vi "MonoVu.vi"() -> ()   [LabVIEW 2020]
doc: "Sequence Program with the Message Handling Queue (MHQ) for the National High Magnetic Field Laboratory in Tallahassee, Florida. \nOnce you understand how the programs works, you should be able to modify this program easily. If you have any questions, contact Minseong Lee(ml10k@my.fsu.edu), who first made this program in June, 2015."
uses:
  <vilib>/printing/OpenHTMLReport.llb/Open HTML Report in Browser (String).vi
  <vilib>/Utility/NIReport.llb/NI_ReportGenerationCore.lvlib
panel:
  out "error out":errorcluster
  in  "error\ncheck":bool
  out "macro line":i32
  in  "exec window":bool caption="command window"
  in  "loop stop":bool
  in  "looped command interval (ms)":u32=100
  in  "wait (ms)":u32
  in  "reset error indicator":bool
  out "Error/\nwarning?":bool
  in  "override command error":bool
  in  "platform":u16(ring) items=["Mac", "PC"]
  out "execution count":i32=1
  in  "sequence utility":bool caption="seq\n utility"
  out "macro cmd no":i32=3
  in  "go to \ncurrent":bool
  in  "help":bool caption="Help"
  in  "Magnet PS":u16(ring)=4 items=["Resistive Magnet", "SCM2", "SCM1", "Generic SC power supply", "PPMS"]
  out "Buffer Edit":string[](array[string])
  out "Path":path=path "/Users/Shared/NML Data Acquisition/Monovu/sequence templates/Examples.txt"
  out "Buffer History":string[](array[string])
  in  "NML Data Acquisition VI":string(combo)="NML Data Acquisition-New.vi"
  in  "Skip Button":bool caption="Skip"
  out "latest error":errorcluster={"status"=TRUE, "code"=1004, "source"="Open VI Reference in Run_VI.vi->MonoVu.vi<APPEND>\nTo load a VI into memory with the Open VI Reference function, a path must be wired for the VI Path input.\n\nVI Name: <b>dsfasdf.vdsafisdaf</b>"}
  in  "error in (no error)":errorcluster
  in  "New Button":bool caption="New"
  in  "Program Stop":bool caption="Program \nStop"
  out "Sequence Status":string="Idle"
  in  "Commands":string(tree)="Set Field"
  in  "Sequence":i32[](listbox)=[16] caption="Sequence*"
  in  "Save Button":bool caption="Save"
  in  "Sequence_Stop":bool caption="Stop"
  in  "Pause Button":bool caption="Pause"
  in  "Run Sequence":bool caption="Run"
  in  "Save As Button":bool caption="Save As"
  out "Cursor Position":i32=16
  out "Current Line":i32
  in  "Open Button":bool caption="Open"
  # "Wait between each execution of command.\ne.g.  if the value is 10, and the command is \n'Wait for Temperature', it checks the temperature every 10 msec. It also forces pause between commands."
  # "(see logbook for previous errors)"
  # "(bypass command syntax error)"
  # "1. Each comand in the sequence line is executed repeatedly until a 'go to next line' command is issued by itself or interrupted by the user. \n2. 'go to next line' condition is defined in the VI for each command. \n\nNote\n(1) For commands with timed or conditioned wait, 'go to next line' command will be issued when the certain condition is met.\n(2) For non-wait command (send command to instruments or VI without waiting response), 'go to next line' is executed automatically.\n(3) For example, 'wait for temperature command' executes repeatedly until the temperature condition is met. The visa reference will be open and closed every time it is executed.\n** Exception: 'Wait for VI value' uses a loop to use the VI reference. The loop condition has to be programmatically reset for the user intervention (skip, pause, stop) accordingly."
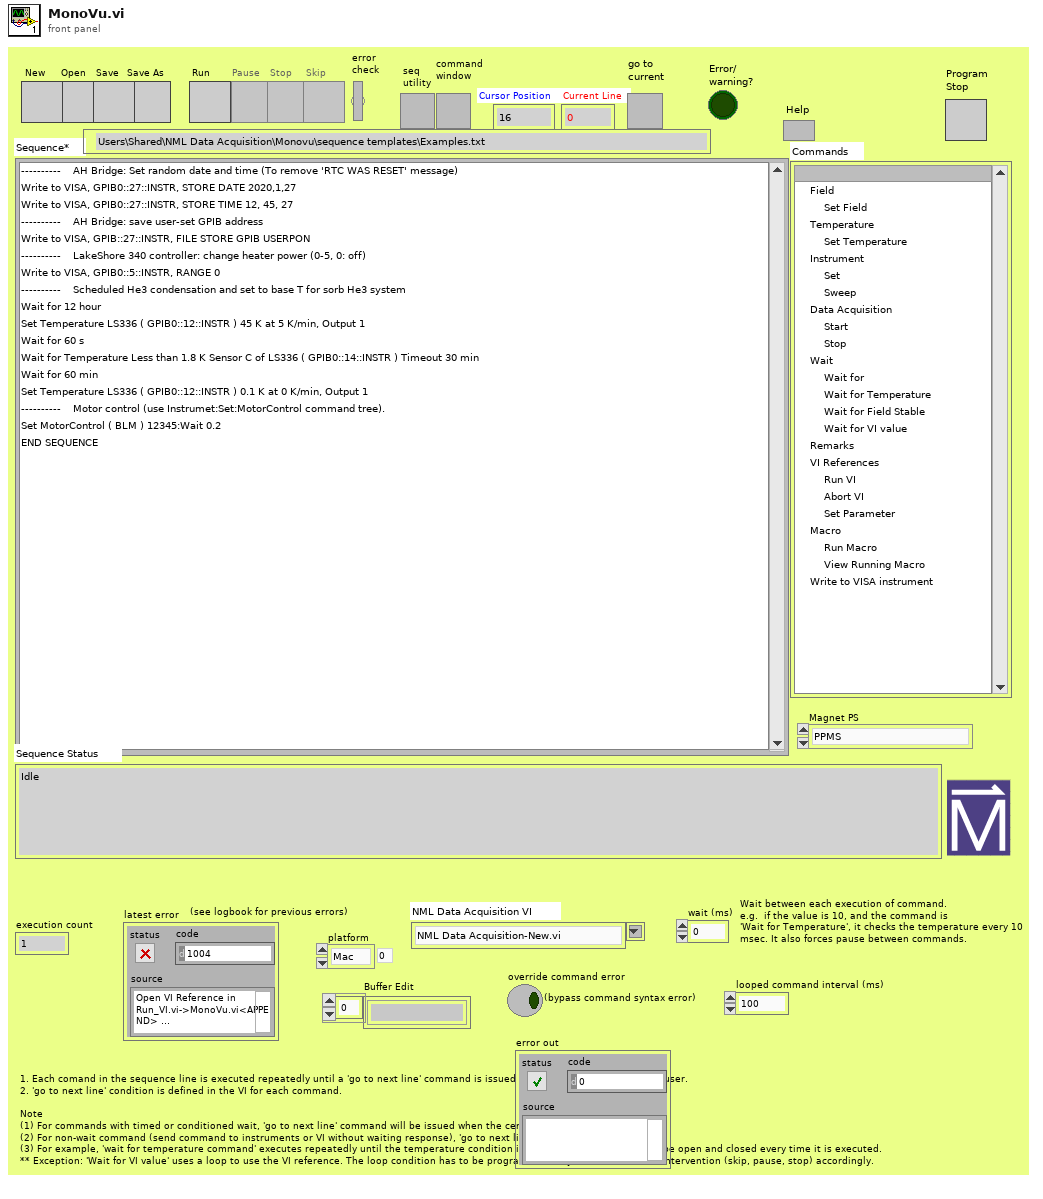
[diagram p1: front panel]
types:
  T1 = cluster{"Sequence_Run":refnum<vi>, "Sequence_Pause":refnum<vi>, "Sequence_Stop":refnum<vi>, "Sequence_Skip":refnum<vi>, "Program Stop":refnum<vi>, "Sequence":refnum<vi>, "NML Data Acquisition VI":refnum<vi>}
  T2 = cluster{"number of line":i32, "Signal":bool, "Command":string, "Sequence Reference":refnum<vi>, "Add or modification":bool}
  T3 = cluster{"No. of command":i32, "Parameters":string[], "Address":refnum<visa-resource-name>, "Boolean":bool, "No. of line":i32, "Initial Time":timestamp, "Current Time":timestamp, "Status":string, "Sequence Ref.":refnum<vi>, "Temp_Check":i32, "Sequence_History":string, "Subsequence":string[]}
  T4 = typedef "Command_Message.ctl" = cluster{"No. of command":i32, "Parameters":string[], "Address":refnum<visa-resource-name>, "Boolean":bool, "No. of line":i32, "Initial Time":timestamp, "Current Time":timestamp, "Status":string, "Sequence Ref.":refnum<vi>, "Temp check":i32, "Sequence_History":string, "Subsequence":string[]}
  T5 = typedef "Button_Reference.ctl" = cluster{"Sequence_Run":refnum<vi>, "Sequence_Pause":refnum<vi>, "Sequence_Stop":refnum<vi>, "Sequence_Skip":refnum<vi>, "Program Stop":refnum<vi>, "Sequence":refnum<vi>, "NML Data Acquisition VI":refnum<vi>}
  T6 = typedef "Command_Queue.ctl" = refnum<queue>
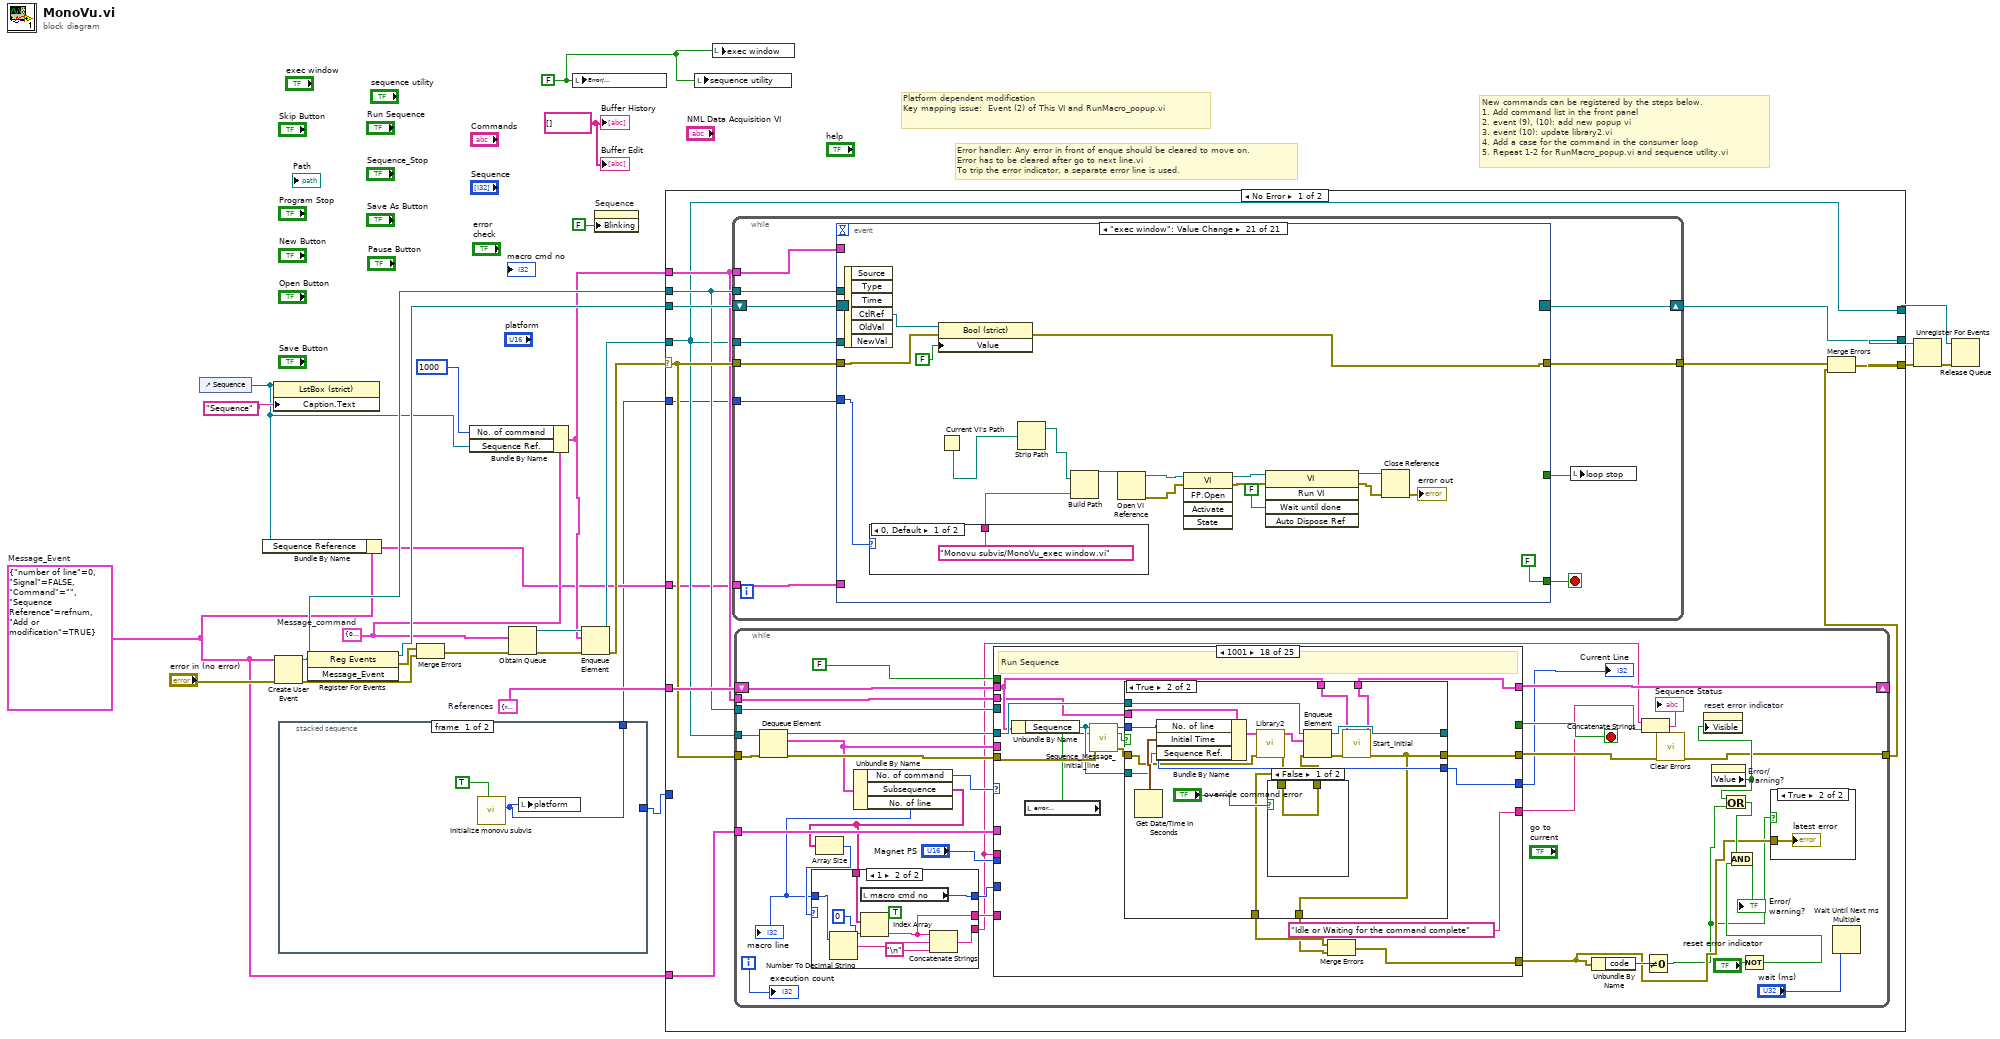
[diagram p0: block diagram]
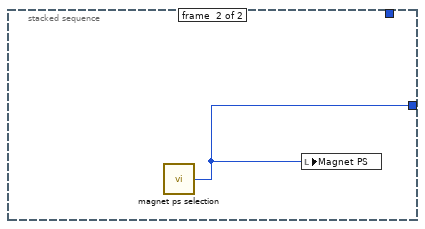
[diagram p2: hidden frame]
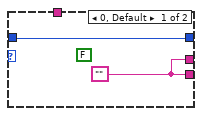
[diagram p4: hidden frame]
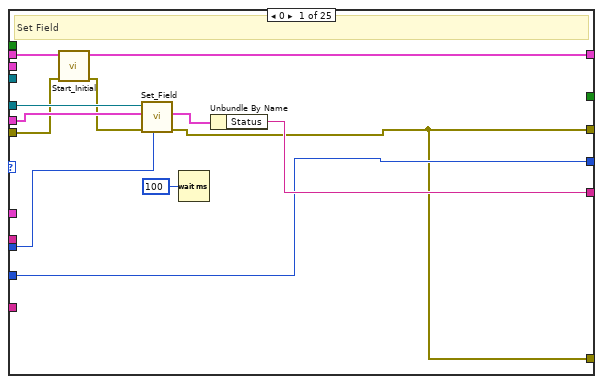
[diagram p5: hidden frame]
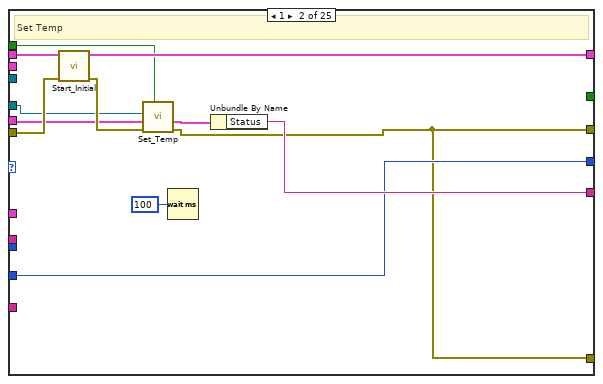
[diagram p6: hidden frame]
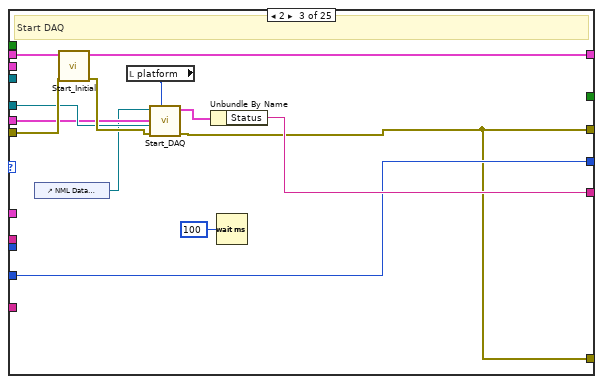
[diagram p7: hidden frame]
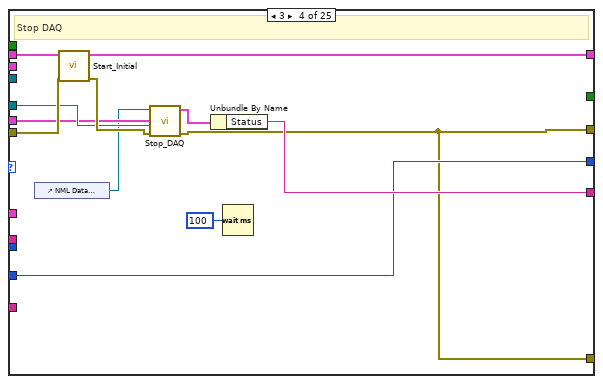
[diagram p8: hidden frame]
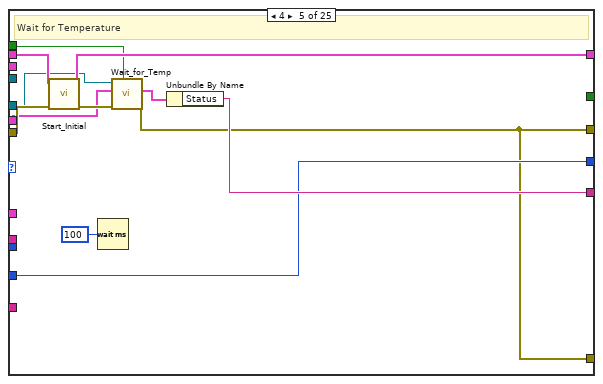
[diagram p9: hidden frame]
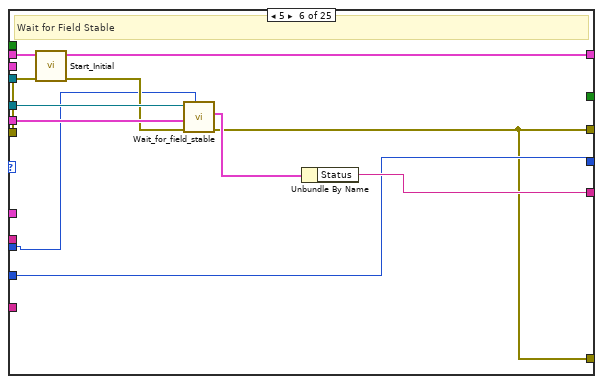
[diagram p10: hidden frame]
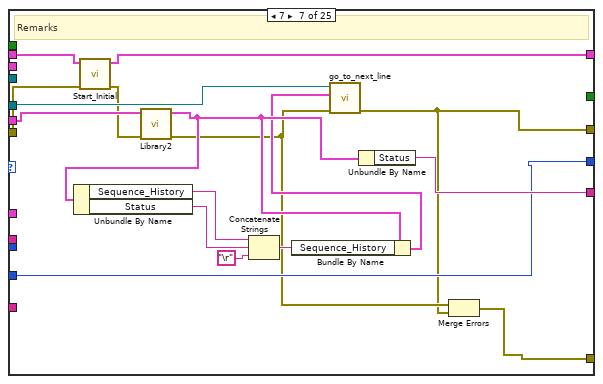
[diagram p11: hidden frame]
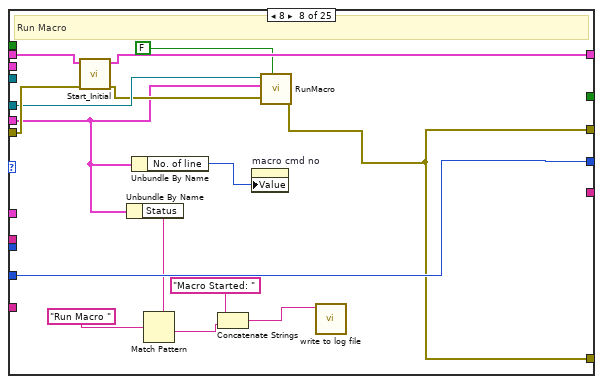
[diagram p12: hidden frame]
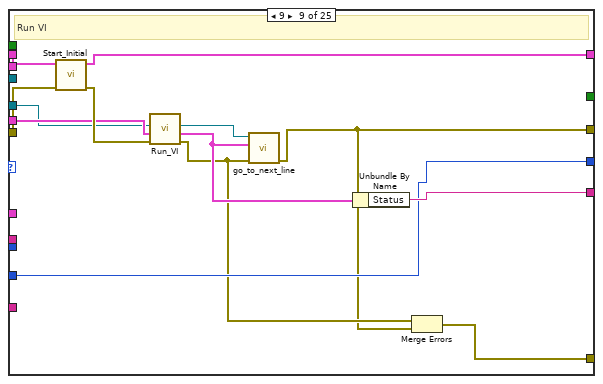
[diagram p13: hidden frame]
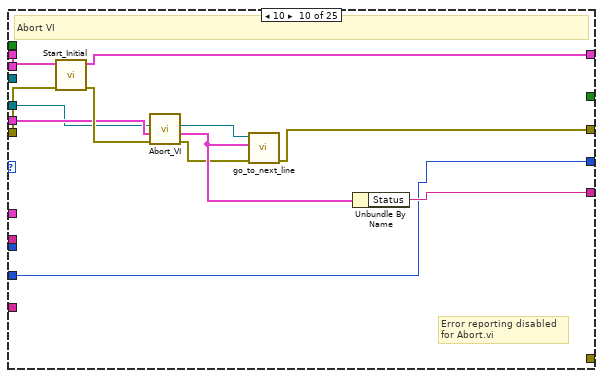
[diagram p14: hidden frame]
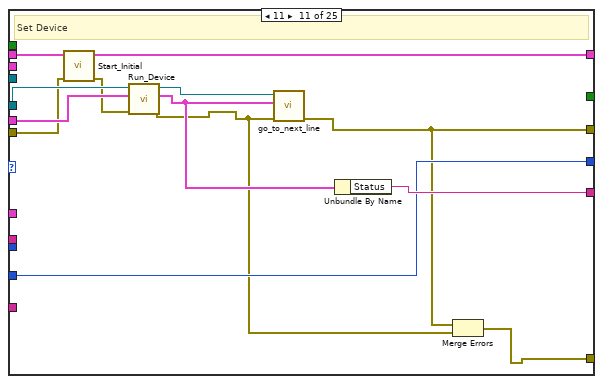
[diagram p15: hidden frame]
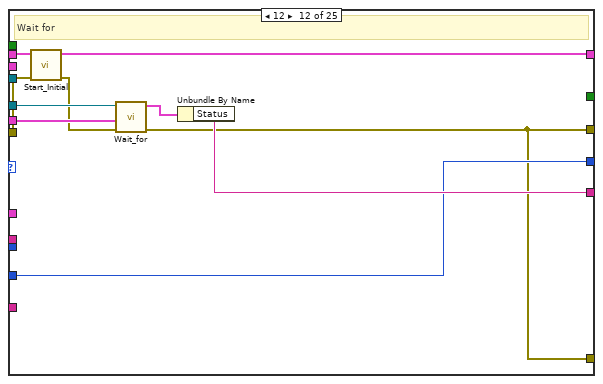
[diagram p16: hidden frame]
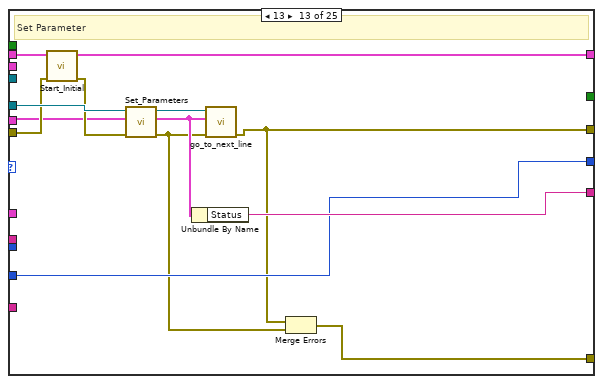
[diagram p17: hidden frame]
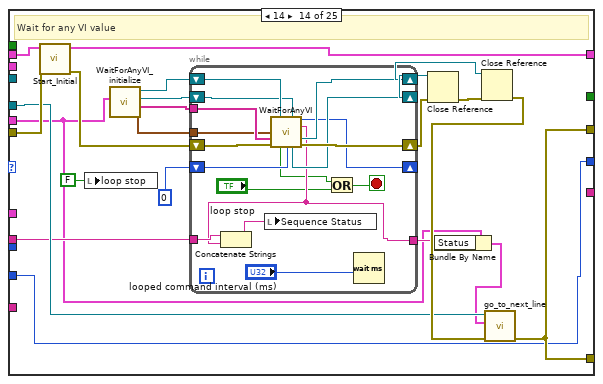
[diagram p18: hidden frame]
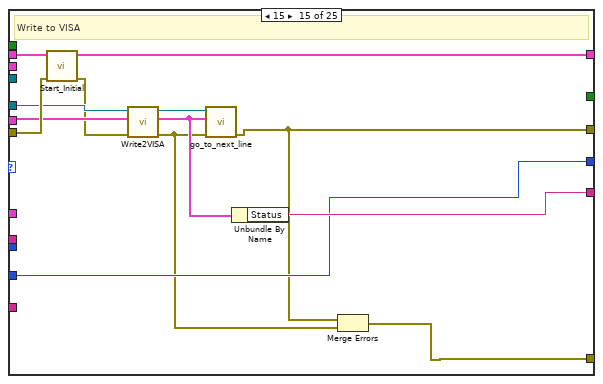
[diagram p19: hidden frame]
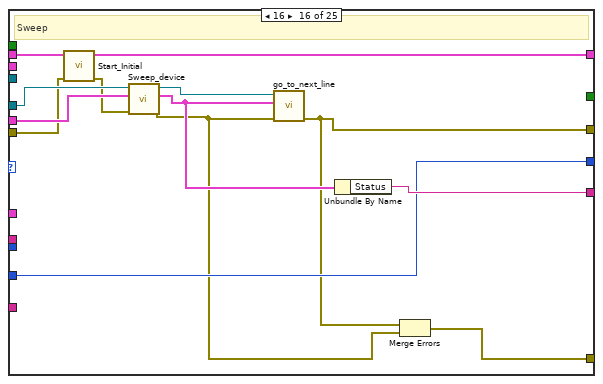
[diagram p20: hidden frame]
diagram:
  w2 = FALSE ("Error?")
  w17 = T1 {"Sequence_Run"=refnum, "Sequence_Pause"=refnum, "Sequence_Stop"=refnum, "Sequence_Skip"=refnum, "Program Stop"=refnum, "Sequence"=refnum, "NML Data Acquisition VI"=refnum}  # References
  w5 = string[] []
  w11 = T2 {"number of line"=0, "Signal"=FALSE, "Command"="", "Sequence Reference"=refnum, "Add or modification"=TRUE}  # Message_Event
  w18 = T3 {"No. of command"=0, "Parameters"=[], "Address"="", "Boolean"=TRUE, "No. of line"=0, "Initial Time"=timestamp(0 s since 1904-01-01), "Current Time"=timestamp(0 s since 1904-01-01), "Status"="", "Sequence Ref."=refnum, "Temp_Check"=0, "Sequence_History"="", "Subsequence"=[]}  # Message_command
  # "Error handler: Any error in front of enque should be cleared to move on.\nError has to be cleared after go to next line.vi\nTo trip the error indicator, a separate error line is used."
  # "Platform dependent modification\nKey mapping issue:  Event (2) of This VI and RunMacro_popup.vi"
  # "New commands can be registered by the steps below.\n1. Add command list in the front panel\n2. event (9), (10): add new popup vi\n3. event (10): update library2.vi \n4. Add a case for the command in the consumer loop\n5. Repeat 1-2 for RunMacro_popup.vi and sequence utility.vi"
  n1 = control-ref of="Sequence"() -> (w6:refnum<vi>)
  n2 = Bundle By Name(cluster=w11, "Sequence Reference"=w6) -> (w10:T2)
  n3 = property class="LstBox (strict)"(reference=w6, "Caption.Text"="Sequence") -> ()  [unwired: 1 in, 2 out]
  n4 = Create User Event(user event datatype=w11, error in="error in (no error)") -> (user event=w23:refnum<user-event>, error out=w25:errorcluster)
  n5 = stacked-sequence {
    tunnel: [_ w30] -> w1
    tunnel: [w28 _] -> w3
    frame #0 {
      n6 = call "Initialize monovu subvis.vi"("auto detect"=TRUE) -> ("platform used"=w28:u16)  [unwired: 9 in, 1 out]
      n7 = local write "platform"(w28) -> ()
    }
    frame #1 {
      n8 = call "magnet ps selection.vi"() -> ("Magnet PS"=w30:u16)  [unwired: 1 in]
      n9 = local write "Magnet PS"(w30) -> ()
    }
  }
  n10 = register-events(w23) -> (reference out=w27:refnum<event-registration>, error out=w24:errorcluster)  [unwired: 2 in]
  n11 = Merge Errors(w24, w25) -> (w8:errorcluster)
  n12 = Bundle By Name(cluster=w18, "No. of command"=1000, "Sequence Ref."=w6) -> (w16:T3)
  n13 = Obtain Queue(element data type=w18, error in (no error)=w8) -> (queue out=w22:refnum<queue>, error out=w20:errorcluster)  [unwired: 3 in, 1 out]
  n14 = local write "Error/\nwarning?"(w2) -> ()
  n15 = Enqueue Element(queue=w22, element=w16, error in (no error)=w20) -> (queue out=w21:refnum<queue>, error out=w19:errorcluster)  [unwired: 1 in, 1 out]
  n16 = property on="Sequence" class="LstBox (strict)"("Blinking"=FALSE) -> ()  [unwired: 2 in, 2 out]
  n17 = case shown="No Error" w19 {
    selector: w19 -> [w40 w1352]
    tunnel: w21 -> [w36 w1350]
    tunnel: [w42 w1352] -> w13
    tunnel: w23 -> [w39 _]
    tunnel: w27 -> [w43 w1351]
    tunnel: w17 -> [w41 _]
    tunnel: w16 -> [w37 _]
    tunnel: w11 -> [w38 _]
    tunnel: [w36 w1350] -> w15
    tunnel: [w34 w1351] -> w14
    tunnel: w10 -> [w32 _]
    tunnel: w1 -> [_ _]
    tunnel: w3 -> [w31 _]
    frame No Error {
      n18 = while {
        tunnel: w36 -> [w481]
        tunnel: w39 -> [w480]
        tunnel: w40 -> [w479]
        tunnel: [w478] -> w35
        tunnel: w37 -> [w477]
        shift-right: [w476] -> w34
        shift-left: w43 -> [w483]
        tunnel: w32 -> [w475]
        tunnel: w31 -> [w474]
        stop <- w482 stop-if-true
        # "Event_Handler"
        n19 = event shown="[20] \"exec window\": Value Change" {
          selector: w483 -> [_ _ _ _ _ _ _ _ _ _ _ _ _ _ _ _ _ _ _ _ _]
          dyn-events: [_ _ _ _ _ _ _ _ _ _ _ _ _ _ _ _ _ _ _ _ _] -> w476
          timeout: _ -> [_ _ _ _ _ _ _ _ _ _ _ _ _ _ _ _ _ _ _ _ _]
          tunnel: [FALSE ("NewVal") FALSE ("NewVal") FALSE ("NewVal") FALSE ("NewVal") FALSE ("NewVal") FALSE ("NewVal") FALSE ("NewVal") FALSE ("NewVal") FALSE ("NewVal") FALSE ("NewVal") FALSE ("NewVal") FALSE ("NewVal") FALSE ("NewVal") FALSE ("NewVal") FALSE ("NewVal") FALSE ("NewVal") w1306 FALSE ("NewVal") TRUE ("NewVal") _ FALSE ("NewVal")] -> w482
          tunnel: w481 -> [w487 _ _ _ _ _ _ _ _ _ _ _ w1248 _ w1285 w1300 w1301 w1309 _ _ _]
          tunnel: w480 -> [w491 _ w675 w803 _ _ _ _ _ w978 w1107 _ _ _ _ _ _ _ _ _ _]
          tunnel: w479 -> [w490 w511 w676 w805 w835 w873 w887 w915 w942 w980 w1116 w1237 w1247 _ w1283 w1299 w1302 w1310 w1316 w1325 w1345]
          tunnel: [w486 w510 w674 w804 w834 w871 w886 w914 w941 w974 w1103 w1237 w1243 _ w1288 w1295 w1307 w1314 w1316 w1323 w1344] -> w478
          tunnel: w477 -> [w488 w509 _ _ _ _ _ _ _ _ w1118 _ w1246 _ w1289 w1298 w1305 w1313 _ _ _]
          tunnel: w475 -> [_ _ w677 w802 _ _ _ _ _ w972 w1108 _ _ _ _ _ _ _ _ _ _]
          tunnel: w474 -> [_ _ w671 _ _ _ _ _ _ w976 w1098 _ _ _ _ _ _ _ _ w1328 w1330]
          tunnel: [_ _ _ _ _ _ _ _ _ _ _ _ w1241 _ TRUE ("loop stop") TRUE ("loop stop") _ _ _ _ _] -> w473
          event "Run Sequence": Value Change {
            n20 = event-data() -> ("NewVal"=w489:bool)  [unwired: 1 in]
            n21 = case shown="True" w489 {
              tunnel: w491 -> [_ _]
              tunnel: w490 -> [w492 w496]
              tunnel: w488 -> [_ w499]
              tunnel: w487 -> [w493 w500]
              tunnel: [w493 w495] -> _
              tunnel: [w492 w494] -> w486
              frame False {
              }
              frame True {
                n22 = Bundle By Name(cluster=w499, "No. of command"=1001) -> (w497:T3)
                n23 = Enqueue Element At Opposite End(queue=w500, element=w497, error in (no error)=w496) -> (queue out=w495:refnum<queue>, error out=w494:errorcluster)  [unwired: 1 in, 1 out]
              }
            }
            n24 = call "write to log file.vi"("input"="Run button pressed") -> ()  [unwired: 9 in, 1 out]
          }
          event User Event {
            n25 = event-data() -> ("number of line"=w508:i32, "Command"=w502:string, "Signal"=w506:bool, "Sequence Reference"=w505:refnum<vi>, "Add or modification"=w504:bool)  [unwired: 1 in]
            n26 = local read "Buffer History"() -> (w503:string[])
            n27 = local read "Buffer Edit"() -> (w501:string[])
            n28 = case shown="\"Undo\"" w502 {
              selector: w502 -> [_ _ _ _ _ w627]
              tunnel: w511 -> [w515 w547 w579 w602 w625 w635]
              tunnel: [w513 w538 w570 w598 w611 w634] -> w510
              tunnel: w509 -> [_ _ _ _ _ w633]
              tunnel: w508 -> [_ _ _ _ _ w632]
              tunnel: w506 -> [_ _ _ _ _ w631]
              tunnel: w505 -> [w512 w548 w580 w603 w626 w630]
              tunnel: w504 -> [_ _ _ _ _ w629]
              tunnel: w503 -> [w514 w543 w575 _ w617 w628]
              tunnel: w501 -> [_ _ _ _ w620 _]
              frame "Undo" {
                n29 = Index Array(array=w514, index=0) -> (element=w522:string)
                n30 = Unflatten From String(type=w514, binary string=w522, error in (no error)=w515) -> (value=w521:string[], error out=w520:errorcluster)  [unwired: 2 in, 1 out]
                n31 = property on="Property Node" class="LstBox (strict)"(reference=w512, error in=w520, "Item Names"=w521) -> (error out=w516:errorcluster)  [unwired: 1 out]
                n32 = Delete From Array(array=w514, length=1, index=0) -> (array with subset deleted=w517:string[])  [unwired: 1 out]
                n33 = property on="Buffer History" class="Arr (strict)"(error in=w516, "Val(Sgnl)"=w517) -> (error out=w513:errorcluster)  [unwired: 1 in, 1 out]
              }
              frame "Cut" {
                n34 = property on="Property Node" class="LstBox (strict)"(reference=w548, error in=w547) -> (reference out=w545:refnum<vi>, error out=w544:errorcluster, "Item Names"=w528:string[], "Value"=w524:i32[])
                n35 = Array Size(array=w524) -> (size(s)=w536:i32)
                n36 = Index Array(array=w524, index=0) -> (element=w535:i32)
                n37 = Delete From Array(array=w528, length=w536, index=w535) -> (deleted portion=w526:string[], array with subset deleted=w529:string[])
                n38 = Array Size(array=w526) -> (size(s)=w534:i32)
                n39 = Decrement(x=w534) -> (x-1=w533:i32)
                n40 = Index Array(array=w526, index=w533) -> (element=w531:string)
                n41 = Equal?(x=w531, y="END SEQUENCE") -> (x = y?=w530:bool)
                n42 = case shown="True" w530 {
                  tunnel: w528 -> [_ w556]
                  tunnel: w536 -> [_ w555]
                  tunnel: w535 -> [_ w553]
                  tunnel: [w550 w552] -> w527
                  tunnel: w529 -> [w550 _]
                  tunnel: w526 -> [w549 _]
                  tunnel: [w549 w551] -> w525
                  frame False {
                  }
                  frame True {
                    n43 = Decrement(x=w555) -> (x-1=w554:i32)
                    n44 = Delete From Array(array=w556, length=w554, index=w553) -> (deleted portion=w551:string[], array with subset deleted=w552:string[])
                  }
                }
                n45 = Flatten To String(anything=w527, error in (no error)=w544) -> (data string=w541:string, error out=w540:errorcluster)  [unwired: 2 in, 1 out]
                n46 = property on="Property Node" class="LstBox (strict)"(reference=w545, error in=w540, "Item Names"=w527, "Val(Sgnl)"=w524) -> (error out=w539:errorcluster)  [unwired: 1 out]
                n47 = Insert Into Array(array=w543, index=0, new element=w541) -> (w537:string[])
                n48 = property on="Buffer History" class="Arr (strict)"(error in=w539, "Val(Sgnl)"=w537) -> (error out=w538:errorcluster)  [unwired: 1 in, 1 out]
                n49 = local write "Buffer Edit"(w525) -> ()
              }
              frame "Delete" {
                n50 = property on="Property Node" class="LstBox (strict)"(reference=w580, error in=w579) -> (reference out=w577:refnum<vi>, error out=w576:errorcluster, "Item Names"=w562:string[], "Value"=w557:i32[])
                n51 = Array Size(array=w557) -> (size(s)=w561:i32)
                n52 = Index Array(array=w557, index=0) -> (element=w560:i32)
                n53 = Delete From Array(array=w562, length=w561, index=w560) -> (deleted portion=w568:string[], array with subset deleted=w559:string[])
                n54 = Array Size(array=w568) -> (size(s)=w564:i32)
                n55 = Decrement(x=w564) -> (x-1=w563:i32)
                n56 = Index Array(array=w568, index=w563) -> (element=w567:string)
                n57 = Equal?(x=w567, y="END SEQUENCE") -> (x = y?=w565:bool)
                n58 = case shown="True" w565 {
                  tunnel: w562 -> [_ w586]
                  tunnel: w561 -> [_ w585]
                  tunnel: w560 -> [_ w583]
                  tunnel: [w581 w582] -> w558
                  tunnel: w559 -> [w581 _]
                  frame False {
                  }
                  frame True {
                    n59 = Decrement(x=w585) -> (x-1=w584:i32)
                    n60 = Delete From Array(array=w586, length=w584, index=w583) -> (array with subset deleted=w582:string[])  [unwired: 1 out]
                  }
                }
                n61 = Flatten To String(anything=w558, error in (no error)=w576) -> (data string=w573:string, error out=w572:errorcluster)  [unwired: 2 in, 1 out]
                n62 = property on="Property Node" class="LstBox (strict)"(reference=w577, error in=w572, "Item Names"=w558, "Val(Sgnl)"=w557) -> (error out=w571:errorcluster)  [unwired: 1 out]
                n63 = Insert Into Array(array=w575, index=0, new element=w573) -> (w569:string[])
                n64 = property on="Buffer History" class="Arr (strict)"(error in=w571, "Val(Sgnl)"=w569) -> (error out=w570:errorcluster)  [unwired: 1 in, 1 out]
              }
              frame "Copy" {
                n65 = property on="Property Node" class="LstBox (strict)"(reference=w603, error in=w602) -> (reference out=w600:refnum<vi>, error out=w599:errorcluster, "Item Names"=w588:string[], "Value"=w587:i32[])
                n66 = Array Size(array=w587) -> (size(s)=w592:i32)
                n67 = Index Array(array=w587, index=0) -> (element=w591:i32)
                n68 = Array Subset(array=w588, index=w591, length=w592) -> (w590:string[])
                n69 = Array Size(array=w590) -> (size(s)=w597:i32)
                n70 = Decrement(x=w597) -> (x-1=w596:i32)
                n71 = property on="Property Node" class="LstBox (strict)"(reference=w600, error in=w599, "Item Names"=w588, "Val(Sgnl)"=w587) -> (error out=w598:errorcluster)  [unwired: 1 out]
                n72 = Index Array(array=w590, index=w596) -> (element=w595:string)
                n73 = Equal?(x=w595, y="END SEQUENCE") -> (x = y?=w593:bool)
                n74 = case shown="True" w593 {
                  tunnel: w592 -> [_ w609]
                  tunnel: w591 -> [_ w607]
                  tunnel: [w604 w605] -> w589
                  tunnel: w590 -> [w604 _]
                  tunnel: w588 -> [_ w606]
                  frame False {
                  }
                  frame True {
                    n75 = Decrement(x=w609) -> (x-1=w608:i32)
                    n76 = Delete From Array(array=w606, length=w608, index=w607) -> (deleted portion=w605:string[])  [unwired: 1 out]
                  }
                }
                n77 = local write "Buffer Edit"(w589) -> ()
              }
              frame "Paste" {
                n78 = property on="Property Node" class="LstBox (strict)"(reference=w626, error in=w625) -> (reference out=w623:refnum<vi>, error out=w614:errorcluster, "Item Names"=w621:string[], "Value"=w610:i32[])
                n79 = Index Array(array=w610, index=0) -> (element=w622:i32)
                n80 = Insert Into Array(array=w621, index=w622, new element=w620) -> (w618:string[])
                n81 = Flatten To String(anything=w618, error in (no error)=w614) -> (data string=w619:string, error out=w613:errorcluster)  [unwired: 2 in, 1 out]
                n82 = property on="Property Node" class="LstBox (strict)"(reference=w623, error in=w613, "Item Names"=w618, "Val(Sgnl)"=w610) -> (error out=w612:errorcluster)  [unwired: 1 out]
                n83 = Insert Into Array(array=w617, index=0, new element=w619) -> (w615:string[])
                n84 = property on="Buffer History" class="Arr (strict)"(error in=w612, "Val(Sgnl)"=w615) -> (error out=w611:errorcluster)  [unwired: 1 in, 1 out]
              }
              frame Default {
                n85 = case shown="True" w629 {
                  tunnel: w635 -> [w652 w669]
                  tunnel: [w637 w654] -> w634
                  tunnel: w633 -> [_ _]
                  tunnel: w632 -> [_ _]
                  tunnel: w631 -> [_ _]
                  tunnel: w630 -> [w651 w668]
                  tunnel: w627 -> [w650 w667]
                  tunnel: w628 -> [w649 w666]
                  frame True {
                    n86 = property class="LstBox (strict)"(reference=w651, error in=w652) -> (reference out=w646:refnum<vi>, error out=w641:errorcluster, "Item Names"=w643:string[], "Value"=w636:i32[])
                    n87 = Index Array(array=w636, index=0) -> (element=w647:i32)
                    n88 = Flatten To String(anything=w643, error in (no error)=w641) -> (data string=w644:string, error out=w642:errorcluster)  [unwired: 2 in, 1 out]
                    n89 = Insert Into Array(array=w643, index=w647, new element=w650) -> (w645:string[])
                    n90 = property class="LstBox (strict)"(reference=w646, error in=w642, "Item Names"=w645, "Value"=w636) -> (error out=w638:errorcluster)  [unwired: 1 out]
                    n91 = Insert Into Array(array=w649, index=0, new element=w644) -> (w639:string[])
                    n92 = property on="Buffer History" class="Arr (strict)"(error in=w638, "Val(Sgnl)"=w639) -> (error out=w637:errorcluster)  [unwired: 1 in, 1 out]
                  }
                  frame False {
                    n93 = property class="LstBox (strict)"(reference=w668, error in=w669) -> (reference out=w663:refnum<vi>, error out=w659:errorcluster, "Item Names"=w660:string[], "Value"=w653:i32[])
                    n94 = Index Array(array=w653, index=0) -> (element=w664:i32)
                    n95 = Flatten To String(anything=w660, error in (no error)=w659) -> (data string=w662:string, error out=w658:errorcluster)  [unwired: 2 in, 1 out]
                    n96 = Replace Array Subset(array=w660, new element=w667, index=w664) -> (w661:string[])
                    n97 = property class="LstBox (strict)"(reference=w663, error in=w658, "Item Names"=w661) -> (error out=w656:errorcluster)  [unwired: 1 out]
                    n98 = Insert Into Array(array=w666, index=0, new element=w662) -> (w655:string[])
                    n99 = property on="Buffer History" class="Arr (strict)"(error in=w656, "Val(Sgnl)"=w655) -> (error out=w654:errorcluster)  [unwired: 1 in, 1 out]
                  }
                }
              }
            }
          }
          event "Sequence": Key Down {
            # "PC:\nDelete:  83\nundo: 44\ncut: 45\ncopy: 46\npaste: 47"
            # "Mac:\nDelete:  117\nundo: 6\ncut: 7\ncopy: 8\npaste: 9"
            n100 = event-data() -> ("ScanCode"=w678:i16, "PlatMods.Ctrl"=w672:bool, "PlatMods.Shift"=w670:bool)  [unwired: 1 in]
            n101 = case shown="0, Default" w671 {
              tunnel: w678 -> [w684 w745]
              tunnel: w677 -> [w683 w744]
              tunnel: w676 -> [w682 w743]
              tunnel: w675 -> [w681 w742]
              tunnel: [w680 w741] -> w674
              tunnel: w672 -> [_ w740]
              tunnel: w670 -> [w679 _]
              frame 1 {
                n102 = case shown="0, Default" w684 {
                  tunnel: w683 -> [_ w690 w693 w705 w717 w729]
                  tunnel: w682 -> [w685 w688 w695 w707 w719 w731]
                  tunnel: w681 -> [_ w687 w692 w704 w716 w728]
                  tunnel: [w685 w686 w694 w706 w718 w730] -> w680
                  tunnel: w679 -> [_ _ w696 w708 w720 w732]
                  frame 0, Default {
                  }
                  frame 83 {
                    n103 = Bundle By Name(cluster=w690, "Command"="Delete") -> (w689:T2)
                    n104 = Generate User Event(user event=w687, event data cluster=w689, error in=w688) -> (error out=w686:errorcluster)  [unwired: 1 in, 1 out]
                  }
                  frame 44 {
                    n105 = case shown="True" w696 {
                      tunnel: w695 -> [w697 w699]
                      tunnel: [w697 w701] -> w694
                      tunnel: w693 -> [_ w700]
                      tunnel: w692 -> [_ w698]
                      frame False {
                      }
                      frame True {
                        n106 = Bundle By Name(cluster=w700, "Command"="Undo") -> (w702:T2)
                        n107 = Generate User Event(user event=w698, event data cluster=w702, error in=w699) -> (error out=w701:errorcluster)  [unwired: 1 in, 1 out]
                      }
                    }
                  }
                  frame 45 {
                    n108 = case shown="True" w708 {
                      tunnel: w707 -> [w709 w711]
                      tunnel: [w709 w713] -> w706
                      tunnel: w705 -> [_ w712]
                      tunnel: w704 -> [_ w710]
                      frame False {
                      }
                      frame True {
                        n109 = Bundle By Name(cluster=w712, "Command"="Cut") -> (w714:T2)
                        n110 = Generate User Event(user event=w710, event data cluster=w714, error in=w711) -> (error out=w713:errorcluster)  [unwired: 1 in, 1 out]
                      }
                    }
                  }
                  frame 46 {
                    n111 = case shown="True" w720 {
                      tunnel: w719 -> [w721 w723]
                      tunnel: [w721 w725] -> w718
                      tunnel: w717 -> [_ w724]
                      tunnel: w716 -> [_ w722]
                      frame False {
                      }
                      frame True {
                        n112 = Bundle By Name(cluster=w724, "Command"="Copy") -> (w726:T2)
                        n113 = Generate User Event(user event=w722, event data cluster=w726, error in=w723) -> (error out=w725:errorcluster)  [unwired: 1 in, 1 out]
                      }
                    }
                  }
                  frame 47 {
                    n114 = case shown="True" w732 {
                      tunnel: w731 -> [w733 w735]
                      tunnel: [w733 w737] -> w730
                      tunnel: w729 -> [_ w736]
                      tunnel: w728 -> [_ w734]
                      frame False {
                      }
                      frame True {
                        n115 = Bundle By Name(cluster=w736, "Command"="Paste") -> (w738:T2)
                        n116 = Generate User Event(user event=w734, event data cluster=w738, error in=w735) -> (error out=w737:errorcluster)  [unwired: 1 in, 1 out]
                      }
                    }
                  }
                }
              }
              frame 0, Default {
                n117 = case shown="0, Default" w745 {
                  tunnel: w744 -> [_ w751 w754 w766 w778 w790]
                  tunnel: w743 -> [w746 w749 w756 w768 w780 w792]
                  tunnel: w742 -> [_ w748 w753 w765 w777 w789]
                  tunnel: [w746 w747 w755 w767 w779 w791] -> w741
                  tunnel: w740 -> [_ _ w757 w769 w781 w793]
                  frame 0, Default {
                  }
                  frame 117 {
                    n118 = Bundle By Name(cluster=w751, "Command"="Delete") -> (w750:T2)
                    n119 = Generate User Event(user event=w748, event data cluster=w750, error in=w749) -> (error out=w747:errorcluster)  [unwired: 1 in, 1 out]
                  }
                  frame 6 {
                    n120 = case shown="True" w757 {
                      tunnel: w756 -> [w758 w760]
                      tunnel: [w758 w762] -> w755
                      tunnel: w754 -> [_ w761]
                      tunnel: w753 -> [_ w759]
                      frame False {
                      }
                      frame True {
                        n121 = Bundle By Name(cluster=w761, "Command"="Undo") -> (w763:T2)
                        n122 = Generate User Event(user event=w759, event data cluster=w763, error in=w760) -> (error out=w762:errorcluster)  [unwired: 1 in, 1 out]
                      }
                    }
                  }
                  frame 7 {
                    n123 = case shown="True" w769 {
                      tunnel: w768 -> [w770 w772]
                      tunnel: [w770 w774] -> w767
                      tunnel: w766 -> [_ w773]
                      tunnel: w765 -> [_ w771]
                      frame False {
                      }
                      frame True {
                        n124 = Bundle By Name(cluster=w773, "Command"="Cut") -> (w775:T2)
                        n125 = Generate User Event(user event=w771, event data cluster=w775, error in=w772) -> (error out=w774:errorcluster)  [unwired: 1 in, 1 out]
                      }
                    }
                  }
                  frame 8 {
                    n126 = case shown="True" w781 {
                      tunnel: w780 -> [w782 w784]
                      tunnel: [w782 w786] -> w779
                      tunnel: w778 -> [_ w785]
                      tunnel: w777 -> [_ w783]
                      frame False {
                      }
                      frame True {
                        n127 = Bundle By Name(cluster=w785, "Command"="Copy") -> (w787:T2)
                        n128 = Generate User Event(user event=w783, event data cluster=w787, error in=w784) -> (error out=w786:errorcluster)  [unwired: 1 in, 1 out]
                      }
                    }
                  }
                  frame 9 {
                    n129 = case shown="True" w793 {
                      tunnel: w792 -> [w794 w796]
                      tunnel: [w794 w798] -> w791
                      tunnel: w790 -> [_ w797]
                      tunnel: w789 -> [_ w795]
                      frame False {
                      }
                      frame True {
                        n130 = Bundle By Name(cluster=w797, "Command"="Paste") -> (w799:T2)
                        n131 = Generate User Event(user event=w795, event data cluster=w799, error in=w796) -> (error out=w798:errorcluster)  [unwired: 1 in, 1 out]
                      }
                    }
                  }
                }
              }
            }
          }
          event "Sequence": Shortcut Menu Selection (User) {
            n132 = event-data() -> ("ItemTag"=w806:string)  [unwired: 1 in]
            n133 = case shown="\"Paste\"" w806 {
              selector: w806 -> [_ w811 w817 w823 w829]
              tunnel: w805 -> [w807 w809 w815 w821 w827]
              tunnel: [w807 w808 w814 w820 w826] -> w804
              tunnel: w803 -> [_ w813 w819 w825 w831]
              tunnel: w802 -> [_ w812 w818 w824 w830]
              frame Default {
              }
              frame "Undo" {
                n134 = Bundle By Name(cluster=w812, "Command"=w811) -> (w810:T2)
                n135 = Generate User Event(user event=w813, event data cluster=w810, error in=w809) -> (error out=w808:errorcluster)  [unwired: 1 in, 1 out]
              }
              frame "Cut" {
                n136 = Bundle By Name(cluster=w818, "Command"=w817) -> (w816:T2)
                n137 = Generate User Event(user event=w819, event data cluster=w816, error in=w815) -> (error out=w814:errorcluster)  [unwired: 1 in, 1 out]
              }
              frame "Copy" {
                n138 = Bundle By Name(cluster=w824, "Command"=w823) -> (w822:T2)
                n139 = Generate User Event(user event=w825, event data cluster=w822, error in=w821) -> (error out=w820:errorcluster)  [unwired: 1 in, 1 out]
              }
              frame "Paste" {
                n140 = Bundle By Name(cluster=w830, "Command"=w829) -> (w828:T2)
                n141 = Generate User Event(user event=w831, event data cluster=w828, error in=w827) -> (error out=w826:errorcluster)  [unwired: 1 in, 1 out]
              }
            }
          }
          event "New Button": Value Change {
            n142 = event-data() -> ("NewVal"=w836:bool, "CtlRef"=w833:refnum<vi>)  [unwired: 1 in]
            n143 = case shown="True" w836 {
              tunnel: w835 -> [w837 w853]
              tunnel: [w837 w845] -> w834
              tunnel: w833 -> [_ w848]
              frame False {
              }
              frame True {
                n144 = property on="Sequence" class="LstBox (strict)"(error in=w853) -> (error out=w844:errorcluster, "Caption.Text"=w852:string, "Item Names"=w849:string[])  [unwired: 1 in, 1 out]
                n145 = property on="Buffer History" class="Arr (strict)"(error in=w844) -> (error out=w843:errorcluster, "Value"=w842:string[])  [unwired: 1 in, 1 out]
                n146 = Equal?(x=w852, y="Sequence*") -> (x = y?=w850:bool)
                n147 = case shown="False" w850 {
                  tunnel: w843 -> [w858 w869]
                  tunnel: w849 -> [_ w870]
                  tunnel: [w859 w864] -> w841
                  tunnel: w848 -> [w857 w863]
                  tunnel: [w857 w863] -> w847
                  tunnel: w842 -> [_ w861]
                  tunnel: [string[] [] ("Buffer out") w860] -> w839
                  frame False {
                    n148 = property on="Sequence" class="LstBox (strict)"(error in=w858, "Item Names"=string[] ["END SEQUENCE"], "Caption.Text"="Sequence") -> (error out=w859:errorcluster)  [unwired: 1 in, 1 out]
                  }
                  frame True {
                    n149 = property on="Path" class="Path"(error in=w869) -> (error out=w868:errorcluster, "Value"=w867:path)  [unwired: 1 in, 1 out]
                    n150 = call "New_File.vi"("error in (no error)"=w868, "Path"=w867, "Buffer in"=w861, "Sequence in"=w870) -> ("error out"=w866:errorcluster, "Sequence Caption"=w862:string, "Buffer out"=w860:string[], "Sequence_out"=w865:string[])  [unwired: 4 in]
                    n151 = property on="Sequence" class="LstBox (strict)"(error in=w866, "Item Names"=w865, "Caption.Text"=w862) -> (error out=w864:errorcluster)  [unwired: 1 in, 1 out]
                  }
                }
                n152 = property on="Buffer History" class="Arr (strict)"(error in=w841, "Value"=w839) -> (error out=w840:errorcluster)  [unwired: 1 in, 1 out]
                n153 = property class="Bool (strict)"(reference=w847, error in=w840, "Value"=FALSE) -> (error out=w845:errorcluster)  [unwired: 1 out]
                n154 = property on="Sequence" class="LstBox (strict)"("Top Row"=0) -> ()  [unwired: 2 in, 2 out]
              }
            }
          }
          event "Buffer History": Value Change {
            n155 = event-data() -> ("NewVal"=w877:string[])  [unwired: 1 in]
            n156 = Array Size(array=w877) -> (size(s)=w876:i32)
            n157 = Equal?(x=w876, y=0) -> (x = y?=w874:bool)
            n158 = case shown="False" w874 {
              tunnel: w873 -> [w879 w882]
              tunnel: [w878 w881] -> w871
              frame True {
                n159 = property on="Sequence" class="LstBox (strict)"(error in=w879, "Caption.Text"="Sequence") -> (error out=w878:errorcluster)  [unwired: 1 in, 1 out]
              }
              frame False {
                n160 = property on="Sequence" class="LstBox (strict)"(error in=w882, "Caption.Text"="Sequence*") -> (error out=w881:errorcluster)  [unwired: 1 in, 1 out]
              }
            }
          }
          event "Open Button": Value Change {
            n161 = event-data() -> ("NewVal"=w888:bool, "CtlRef"=w885:refnum<vi>)  [unwired: 1 in]
            n162 = case shown="True" w888 {
              tunnel: w887 -> [w889 w911]
              tunnel: [w889 w892] -> w886
              tunnel: w885 -> [_ w895]
              frame False {
              }
              frame True {
                n163 = property on="Sequence" class="LstBox (strict)"(error in=w911) -> (error out=w907:errorcluster, "Caption.Text"=w909:string, "Item Names"=w908:string[])  [unwired: 1 in, 1 out]
                n164 = Equal?(x=w909, y="Sequence*") -> (x = y?=w896:bool)
                n165 = property on="Buffer History" class="Arr (strict)"(error in=w907) -> (error out=w905:errorcluster, "Value"=w906:string[])  [unwired: 1 in, 1 out]
                n166 = property on="Path" class="Path"(error in=w905) -> (error out=w903:errorcluster, "Value"=w904:path)  [unwired: 1 in, 1 out]
                n167 = call "Open_File.vi"("Message?"=w896, "Path in"=w904, "error in (no error)"=w903, "Sequence in"=w908, "Buffer in"=w906, "Sequence Caption in"=w909) -> ("error out"=w891:errorcluster, "Sequence out"=w901:string[], "Buffer out"=w899:string[], "Sequence Caption out"=w902:string, "Path out"=w897:path, "top row"=w890:i32)
                n168 = property on="Sequence" class="LstBox (strict)"("Top Row"=w890) -> ()  [unwired: 2 in, 2 out]
                n169 = property on="Sequence" class="LstBox (strict)"(error in=w891, "Item Names"=w901, "Caption.Text"=w902) -> (error out=w900:errorcluster)  [unwired: 1 in, 1 out]
                n170 = property on="Buffer History" class="Arr (strict)"(error in=w900, "Value"=w899) -> (error out=w898:errorcluster)  [unwired: 1 in, 1 out]
                n171 = property on="Path" class="Path"(error in=w898, "Value"=w897) -> (error out=w894:errorcluster)  [unwired: 1 in, 1 out]
                n172 = property class="Bool (strict)"(reference=w895, error in=w894, "Value"=FALSE) -> (error out=w892:errorcluster)  [unwired: 1 out]
              }
            }
          }
          event "Save Button": Value Change {
            n173 = event-data() -> ("NewVal"=w916:bool, "CtlRef"=w913:refnum<vi>)  [unwired: 1 in]
            n174 = case shown="True" w916 {
              tunnel: w915 -> [w917 w934]
              tunnel: [w917 w918] -> w914
              tunnel: w913 -> [_ w921]
              frame False {
              }
              frame True {
                n175 = property on="Path" class="Path"(error in=w934) -> (error out=w933:errorcluster, "Value"=w936:path)  [unwired: 1 in, 1 out]
                n176 = Not Equal?(x=path "", y=w936) -> (x != y?=w937:bool)
                n177 = property on="Buffer History" class="Arr (strict)"(error in=w933) -> (error out=w932:errorcluster, "Value"=w935:string[])  [unwired: 1 in, 1 out]
                n178 = property on="Sequence" class="LstBox (strict)"(error in=w932) -> (error out=w931:errorcluster, "Item Names"=w930:string[], "Caption.Text"=w929:string)  [unwired: 1 in, 1 out]
                n179 = call "Save_File.vi"("Sequence caption in"=w929, "Path?"=w937, "error in (no error)"=w931, "Sequence in"=w930, "Buffer in"=w935, "Path in"=w936) -> ("error out"=w928:errorcluster, "Sequence out"=w924:string[], "Buffer out"=w926:string[], "Path out"=w922:path, "Sequence caption out"=w925:string)  [unwired: 1 in]
                n180 = property on="Buffer History" class="Arr (strict)"(error in=w928, "Value"=w926) -> (error out=w927:errorcluster)  [unwired: 1 in, 1 out]
                n181 = property on="Sequence" class="LstBox (strict)"(error in=w927, "Item Names"=w924, "Caption.Text"=w925) -> (error out=w923:errorcluster)  [unwired: 1 in, 1 out]
                n182 = property on="Path" class="Path"(error in=w923, "Value"=w922) -> (error out=w920:errorcluster)  [unwired: 1 in, 1 out]
                n183 = property class="Bool (strict)"(reference=w921, error in=w920, "Value"=FALSE) -> (error out=w918:errorcluster)  [unwired: 1 out]
              }
            }
          }
          event "Save As Button": Value Change {
            n184 = event-data() -> ("NewVal"=w943:bool, "CtlRef"=w940:refnum<vi>)  [unwired: 1 in]
            n185 = case shown="True" w943 {
              tunnel: w942 -> [w944 w962]
              tunnel: [w944 w946] -> w941
              tunnel: w940 -> [_ w949]
              frame False {
              }
              frame True {
                n186 = property on="Path" class="Path"(error in=w962) -> (error out=w961:errorcluster, "Value"=w964:path)  [unwired: 1 in, 1 out]
                n187 = property on="Buffer History" class="Arr (strict)"(error in=w961) -> (error out=w960:errorcluster, "Value"=w963:string[])  [unwired: 1 in, 1 out]
                n188 = property on="Sequence" class="LstBox (strict)"(error in=w960) -> (error out=w959:errorcluster, "Item Names"=w958:string[], "Caption.Text"=w957:string)  [unwired: 1 in, 1 out]
                n189 = call "Save_File.vi"("Sequence caption in"=w957, "Path?"=FALSE, "error in (no error)"=w959, "Sequence in"=w958, "Buffer in"=w963, "Path in"=w964) -> ("error out"=w956:errorcluster, "Sequence out"=w952:string[], "Buffer out"=w954:string[], "Path out"=w950:path, "Sequence caption out"=w953:string)  [unwired: 1 in]
                n190 = property on="Buffer History" class="Arr (strict)"(error in=w956, "Value"=w954) -> (error out=w955:errorcluster)  [unwired: 1 in, 1 out]
                n191 = property on="Sequence" class="LstBox (strict)"(error in=w955, "Item Names"=w952, "Caption.Text"=w953) -> (error out=w951:errorcluster)  [unwired: 1 in, 1 out]
                n192 = property on="Path" class="Path"(error in=w951, "Value"=w950) -> (error out=w948:errorcluster)  [unwired: 1 in, 1 out]
                n193 = property class="Bool (strict)"(reference=w949, error in=w948, "Value"=FALSE) -> (error out=w946:errorcluster)  [unwired: 1 out]
              }
            }
          }
          event "Commands": Double Click {
            n194 = event-data() -> ("Tag"=w979:string)  [unwired: 1 in]
            n195 = case shown="\"Run VI\"" w979 {
              tunnel: w980 -> [w991 w997 w1003 w1009 w1015 w1021 w1027 w1033 w1039 w1045 w1051 w1057 w1060 w1065 w1073 w1081 w1082 w1087]
              tunnel: [w991 w995 w1000 w1007 w1012 w1018 w1024 w1030 w1036 w1042 w1048 w1054 w1060 w1065 w1070 w1076 w1084 w1090] -> w975
              tunnel: w978 -> [w990 w994 w1001 w1008 w1014 w1020 w1026 w1032 w1038 w1044 w1050 w1056 w1062 w1067 w1072 w1078 _ w1092]
              tunnel: w976 -> [_ _ _ _ _ _ _ _ _ _ _ _ _ _ _ w1079 _ _]
              tunnel: [TRUE ("Cancel") w996 w1002 w1006 w1013 w1019 w1025 w1031 w1037 w1043 w1049 w1055 FALSE ("Signal") FALSE ("Signal") w1071 w1077 _ w1091] -> w967
              tunnel: [w990 w994 w1001 w1008 w1014 w1020 w1026 w1032 w1038 w1044 w1050 w1056 w1062 w1067 w1072 w1078 _ w1092] -> w973
              tunnel: [_ TRUE ("Add or modification") TRUE ("Add or modification") TRUE ("Add or modification") TRUE ("Add or modification") TRUE ("Add or modification") TRUE ("Add or modification") TRUE ("Add or modification") TRUE ("Add or modification") TRUE ("Add or modification") TRUE ("Add or modification") TRUE ("Add or modification") TRUE ("Add or modification") TRUE ("Add or modification") TRUE ("Signal") TRUE ("Signal") _ TRUE ("Add or modification")] -> w971
              tunnel: [_ w993 w998 w1004 w1010 w1016 w1022 w1028 w1034 w1041 w1046 w1052 "Stop" ("Command") "Wait for Field Stable" ("Command") w1068 w1074 _ w1088] -> w969
              frame Default {
              }
              frame "Set Field" {
                n196 = call "SetField_popup.vi"("error in (no error)"=w997) -> ("Output Line command"=w993:string, "Cancel"=w996:bool, "error out"=w995:errorcluster)  [unwired: 5 in]
              }
              frame "Set Temperature" {
                n197 = call "SetTemp_popup.vi"("error in (no error)"=w1003) -> ("error out"=w1000:errorcluster, "Cancel"=w1002:bool, "Output Line Command"=w998:string)  [unwired: 7 in]
              }
              frame "Wait for Temperature" {
                n198 = call "SetWaitForTemp_popup.vi"("error in (no error)"=w1009) -> ("Output Line Command"=w1004:string, "Cancel"=w1006:bool, "error out"=w1007:errorcluster)  [unwired: 7 in]
              }
              frame "Wait for" {
                n199 = call "SetWaitFor_popup.vi"("error in (no error)"=w1015) -> ("error out"=w1012:errorcluster, "Cancel"=w1013:bool, "Output Line Command"=w1010:string)  [unwired: 7 in]
              }
              frame "Start" {
                n200 = call "SetStart_popup.vi"("error in (no error)"=w1021) -> ("Output Line Command"=w1016:string, "Cancel"=w1019:bool, "error out"=w1018:errorcluster)  [unwired: 7 in]
              }
              frame "Remarks" {
                n201 = call "SetRemarks_popup.vi"("error in (no error)"=w1027) -> ("Cancel"=w1025:bool, "Output Line Command"=w1022:string, "error out"=w1024:errorcluster)  [unwired: 7 in]
              }
              frame "Run VI" {
                n202 = call "SetRunVI_popup.vi"("error in (no error)"=w1033) -> ("Cancel"=w1031:bool, "Output Line Command"=w1028:string, "error out"=w1030:errorcluster)  [unwired: 7 in]
              }
              frame "Abort VI" {
                n203 = call "SetAbortVI_popup.vi"("error in (no error)"=w1039) -> ("Cancel"=w1037:bool, "Output Line Command"=w1034:string, "error out"=w1036:errorcluster)  [unwired: 7 in]
              }
              frame "Set Parameter" {
                n204 = call "SetParameter_popup.vi"("error in (no error)"=w1045) -> ("error out"=w1042:errorcluster, "Cancel"=w1043:bool, "Output Line Command"=w1041:string)  [unwired: 7 in]
              }
              frame "Set" {
                n205 = call "SetDevice_popup.vi"("error in (no error)"=w1051) -> ("Cancel"=w1049:bool, "Output Line Command"=w1046:string, "error out"=w1048:errorcluster)  [unwired: 7 in]
              }
              frame "Sweep" {
                n206 = call "SetSweep_popup.vi"("error in (no error)"=w1057) -> ("Cancel"=w1055:bool, "Output Line Command"=w1052:string, "error out"=w1054:errorcluster)  [unwired: 7 in]
              }
              frame "Stop" {
              }
              frame "Wait for Field Stable" {
              }
              frame "Wait for VI value" {
                n207 = call "SetWaitForAnyVI_popup.vi"("error in (no error)"=w1073) -> ("error out"=w1070:errorcluster, "Cancel"=w1071:bool, "Output Line Command"=w1068:string)  [unwired: 7 in]
              }
              frame "Run Macro" {
                n208 = call "RunMacro_popup.vi"("load?"=FALSE, "platform"=w1079, "error in (no error)"=w1081) -> ("Cancel"=w1077:bool, "command out"=w1074:string, "error out"=w1076:errorcluster)  [unwired: 5 in]
              }
              frame "View Running Macro" {
                n209 = vi-ref "RunMacro.vi"() -> (w1086:refnum<vi>)
                n210 = invoke class="VI" method="FP.Open"(reference=w1086, error in=w1082) -> (reference out=w1085:refnum<vi>, error out=w1083:errorcluster)  [unwired: 3 in, 3 out]
                n211 = Close Reference(reference=w1085, error in (no error)=w1083) -> (error out=w1084:errorcluster)
              }
              frame "Write to VISA instrument" {
                n212 = call "WriteVISA_popup.vi"("error in (no error)"=w1087) -> ("Output Line Command"=w1088:string, "Cancel"=w1091:bool, "error out"=w1090:errorcluster)  [unwired: 8 in]
              }
            }
            n213 = local read "error\ncheck"() -> (w965:bool)
            n214 = case shown="True" w965 {
              tunnel: w969 -> [_ w984]
              tunnel: [FALSE ("error") w982] -> w968
              frame False {
              }
              frame True {
                n215 = Build Array(w984) -> (w983:string[])
                n216 = call "sequence util_error check.vi"("Item Names IN"=w983) -> ("error"=w982:bool)  [unwired: 8 in, 1 out]
              }
            }
            n217 = Or(x=w967, y=w968) -> (x .or. y?=w966:bool)
            n218 = Bundle By Name(cluster=w972, "Signal"=w967, "Command"=w969, "Add or modification"=w971) -> (w970:T2)
            n219 = case shown="False" w966 {
              tunnel: w973 -> [w987 _]
              tunnel: w970 -> [w986 _]
              tunnel: [w985 w988] -> w974
              tunnel: w975 -> [_ w988]
              frame False {
                n220 = Generate User Event(user event=w987, event data cluster=w986) -> (error out=w985:errorcluster)  [unwired: 2 in, 1 out]
              }
              frame True {
              }
            }
          }
          event "Sequence": Double Click {
            # "check if the sequence is changed. Returns 'False\"\nIf (1) 'cancel' button pressed \nOR (2) 'ok' button pressed but no value change"
            n221 = event-data() -> ("Row"=w1109:i32)  [unwired: 1 in]
            n222 = Bundle By Name(cluster=w1118, "No. of line"=w1109) -> (w1117:T3)
            n223 = Unbundle By Name(w1108) -> ("Sequence Reference"=w1113:refnum<vi>)
            n224 = call "Library2.vi"("Message_command_in"=w1117, "error in (no error)"=w1116) -> ("Message_command out"=w1115:T4, "error out"=w1112:errorcluster)  [unwired: 7 in]
            n225 = property class="LstBox (strict)"(reference=w1113, error in=w1112) -> (error out=w1111:errorcluster, "Item Names"=w1110:string[])  [unwired: 1 out]
            n226 = Unbundle By Name(w1115) -> ("No. of command"=w1114:i32)
            n227 = local read "error\ncheck"() -> (w1093:bool)
            n228 = Index Array(array=w1110, index=w1109) -> (element=w1099:string)
            n229 = case shown="13" w1114 {
              tunnel: w1111 -> [w1138 w1145 w1152 w1159 w1166 w1173 w1182 w1189 w1196 w1203 w1210 w1217 w1218 w1231 w1235]
              tunnel: w1099 -> [w1137 w1144 w1151 w1158 w1165 w1168 w1181 w1188 w1195 w1202 w1209 w1216 w1222 w1230 _]
              tunnel: w1108 -> [w1135 w1142 w1149 w1156 w1163 w1175 w1179 w1186 w1193 w1200 w1207 w1214 w1224 w1228 w1234]
              tunnel: w1107 -> [w1134 w1141 w1148 w1155 w1162 w1174 w1178 w1185 w1192 w1199 w1206 w1213 w1223 w1227 w1233]
              tunnel: [w1136 w1143 w1150 w1157 w1164 w1170 w1180 w1187 w1194 w1201 w1208 w1211 w1221 w1229 w1235] -> w1104
              tunnel: [w1135 w1142 w1149 w1156 w1163 w1175 w1179 w1186 w1193 w1200 w1207 w1214 w1224 w1228 w1234] -> w1106
              tunnel: [w1134 w1141 w1148 w1155 w1162 w1174 w1178 w1185 w1192 w1199 w1206 w1213 w1223 w1227 w1233] -> w1105
              tunnel: [w1133 w1140 w1147 w1154 w1161 w1171 w1177 w1184 w1191 w1197 w1204 w1212 w1220 w1226 TRUE ("Cancel")] -> w1100
              tunnel: [w1132 w1139 w1146 w1153 w1160 w1172 w1176 w1183 w1190 w1198 w1205 w1215 w1219 w1225 _] -> w1096
              tunnel: w1098 -> [_ _ _ _ _ w1167 _ _ _ _ _ _ _ _ _]
              frame 0 {
                n230 = call "SetField_popup.vi"("error in (no error)"=w1138, "Input Line command"=w1137) -> ("Output Line command"=w1132:string, "Cancel"=w1133:bool, "error out"=w1136:errorcluster)  [unwired: 4 in]
              }
              frame 1 {
                n231 = call "SetTemp_popup.vi"("Input Line Command"=w1144, "error in (no error)"=w1145) -> ("error out"=w1143:errorcluster, "Cancel"=w1140:bool, "Output Line Command"=w1139:string)  [unwired: 6 in]
              }
              frame 2 {
                n232 = call "SetStart_popup.vi"("Input Line Command"=w1151, "error in (no error)"=w1152) -> ("Output Line Command"=w1146:string, "Cancel"=w1147:bool, "error out"=w1150:errorcluster)  [unwired: 6 in]
              }
              frame 4 {
                n233 = call "SetWaitForTemp_popup.vi"("Input Line Command"=w1158, "error in (no error)"=w1159) -> ("Output Line Command"=w1153:string, "Cancel"=w1154:bool, "error out"=w1157:errorcluster)  [unwired: 6 in]
              }
              frame 7 {
                n234 = call "SetRemarks_popup.vi"("Input Line Command"=w1165, "error in (no error)"=w1166) -> ("Cancel"=w1161:bool, "Output Line Command"=w1160:string, "error out"=w1164:errorcluster)  [unwired: 6 in]
              }
              frame 8 {
                n235 = call "RunMacro_popup.vi"("load?"=TRUE, "platform"=w1167, "command in"=w1168, "error in (no error)"=w1173) -> ("Cancel"=w1171:bool, "command out"=w1172:string, "error out"=w1170:errorcluster)  [unwired: 4 in]
              }
              frame 9 {
                n236 = call "SetRunVI_popup.vi"("Input Line Command"=w1181, "error in (no error)"=w1182) -> ("Cancel"=w1177:bool, "Output Line Command"=w1176:string, "error out"=w1180:errorcluster)  [unwired: 6 in]
              }
              frame 10 {
                n237 = call "SetAbortVI_popup.vi"("Input Line Command"=w1188, "error in (no error)"=w1189) -> ("Cancel"=w1184:bool, "Output Line Command"=w1183:string, "error out"=w1187:errorcluster)  [unwired: 6 in]
              }
              frame 11 {
                n238 = call "SetDevice_popup.vi"("Input Line Command"=w1195, "error in (no error)"=w1196) -> ("Cancel"=w1191:bool, "Output Line Command"=w1190:string, "error out"=w1194:errorcluster)  [unwired: 6 in]
              }
              frame 12 {
                n239 = call "SetWaitFor_popup.vi"("Input Line Command"=w1202, "error in (no error)"=w1203) -> ("error out"=w1201:errorcluster, "Cancel"=w1197:bool, "Output Line Command"=w1198:string)  [unwired: 6 in]
              }
              frame 13 {
                n240 = call "SetParameter_popup.vi"("Input Line Command"=w1209, "error in (no error)"=w1210) -> ("error out"=w1208:errorcluster, "Cancel"=w1204:bool, "Output Line Command"=w1205:string)  [unwired: 6 in]
              }
              frame 14 {
                n241 = call "SetWaitForAnyVI_popup.vi"("Input Line Command"=w1216, "error in (no error)"=w1217) -> ("error out"=w1211:errorcluster, "Cancel"=w1212:bool, "Output Line Command"=w1215:string)  [unwired: 6 in]
              }
              frame 15 {
                n242 = call "WriteVISA_popup.vi"("error in (no error)"=w1218, "Input Line Command"=w1222) -> ("Output Line Command"=w1219:string, "Cancel"=w1220:bool, "error out"=w1221:errorcluster)  [unwired: 7 in]
              }
              frame 16 {
                n243 = call "SetSweep_popup.vi"("Input Line Command"=w1230, "error in (no error)"=w1231) -> ("Cancel"=w1226:bool, "Output Line Command"=w1225:string, "error out"=w1229:errorcluster)  [unwired: 6 in]
              }
              frame Default {
              }
            }
            n244 = case shown="False" w1093 {
              tunnel: w1096 -> [_ w1122]
              tunnel: [FALSE ("error") w1120] -> w1097
              frame False {
              }
              frame True {
                n245 = Build Array(w1122) -> (w1121:string[])
                n246 = call "sequence util_error check.vi"("Item Names IN"=w1121) -> ("error"=w1120:bool)  [unwired: 8 in, 1 out]
              }
            }
            n247 = Equal?(x=w1099, y=w1096) -> (x = y?=w1101:bool)
            n248 = Or(x=w1100, y=w1101) -> (x .or. y?=w1095:bool)
            n249 = Or(x=w1095, y=w1097) -> (x .or. y?=w1094:bool)
            n250 = case shown="True" w1094 {
              selector: w1094 -> [w1125 _]
              tunnel: w1106 -> [w1129 _]
              tunnel: w1105 -> [w1127 _]
              tunnel: w1096 -> [w1126 _]
              tunnel: w1104 -> [w1124 w1131]
              tunnel: [w1123 w1131] -> w1103
              frame False {
                n251 = Bundle By Name(cluster=w1129, "Signal"=w1125, "Command"=w1126, "Add or modification"=FALSE) -> (w1128:T2)
                n252 = Generate User Event(user event=w1127, event data cluster=w1128, error in=w1124) -> (error out=w1123:errorcluster)  [unwired: 1 in, 1 out]
              }
              frame True {
              }
            }
          }
          event "Sequence": Value Change {
            n253 = event-data() -> ("NewVal"=w1240:i32[])  [unwired: 1 in]
            n254 = Index Array(array=w1240, index=0) -> (element=→"Cursor Position":i32)
          }
          event "Pause Button": Value Change {
            # "Note: unpause restart the execution line. For example, if it was paused\nduring 'Wait for 1 hr' line, the stopwatch will reset after unpause (waiting\nanother 1 hr). \nFor the subsequence, it restarts the line of the subsequence."
            # "for the looped command, \npause will stop the loop,\nunpause will resume the loop"
            n255 = event-data() -> ("NewVal"=w1245:bool)  [unwired: 1 in]
            n256 = local read "Current Line"() -> (w1244:i32)
            n257 = case shown="True" w1245 {
              tunnel: w1248 -> [w1255 w1265]
              tunnel: w1247 -> [_ w1264]
              tunnel: w1246 -> [w1251 w1263]
              tunnel: w1245 -> [_ w1261]
              tunnel: w1244 -> [w1254 w1260]
              tunnel: [w1253 w1257] -> w1243
              tunnel: [FALSE ("loop stop") TRUE ("loop stop")] -> w1241
              frame False {
                n258 = Decrement(x=w1254) -> (x-1=w1252:i32)
                n259 = Bundle By Name(cluster=w1251, "No. of line"=w1252) -> (w1250:T3)
                n260 = call "go_to_next_line.vi"("Message_command in"=w1250, "Command Queue in"=w1255) -> ("error out"=w1253:errorcluster)  [unwired: 8 in, 1 out]
              }
              frame True {
                n261 = flat-sequence {
                  frame #0 {
                    w1268 = "RunMacro.vi" ("VI Name")
                    n262 = local read "macro line"() -> (w1266:i32)
                    n263 = call "set_control_in_Memory.vi"("Control Name"="restart line", "Value"=w1266, "VI Name"=w1268) -> ()  [unwired: 2 in, 1 out]
                    n264 = call "set_control_in_Memory.vi"("Control Name"="paused?", "Value"=TRUE ("loop stop"), "VI Name"=w1268) -> ()  [unwired: 2 in, 1 out]
                  }
                }
                n265 = Bundle By Name(cluster=w1263, "No. of command"=1002, "Boolean"=w1261, "No. of line"=w1260, "Status"="Pause" ("Sequence status")) -> (w1259:T3)
                n266 = Enqueue Element At Opposite End(queue=w1265, element=w1259, error in (no error)=w1264) -> (error out=w1257:errorcluster)  [unwired: 1 in, 2 out]
              }
            }
          }
          event "go to \ncurrent": Value Change {
            w1277 = 10  # halfline
            n267 = event-data() -> ()  [unwired: 1 in, 1 out]
            n268 = local read "Current Line"() -> (w1278:i32)
            n269 = local read "Sequence"() -> (w1276:i32[])
            n270 = Subtract(x=w1278, y=w1277) -> (x-y=w1272:i32)
            n271 = Replace Array Subset(array=w1276, new element=w1278, index=0) -> (w1274:i32[])
            n272 = local write "Sequence"(w1274) -> ()
            n273 = Max & Min(x=u8 0, y=w1272) -> (max(x,y)=w1271:i32)  [unwired: 1 out]
            n274 = property on="Sequence" class="LstBox (strict)"("Top Row"=w1271) -> ()  [unwired: 2 in, 2 out]
          }
          event "Skip Button": Value Change {
            n275 = event-data() -> ()  [unwired: 1 in, 1 out]
            n276 = Bundle By Name(cluster=w1289, "No. of command"=1004) -> (w1286:T3)
            n277 = Flush Queue(queue=w1285, error in (no error)=w1283) -> (queue out=w1284:refnum<queue>, error out=w1282:errorcluster)  [unwired: 1 out]
            n278 = Enqueue Element At Opposite End(queue=w1284, element=w1286, error in (no error)=w1282) -> (error out=w1288:errorcluster)  [unwired: 1 in, 2 out]
          }
          event "Sequence_Stop": Value Change {
            n279 = event-data() -> ("NewVal"=w1297:bool)  [unwired: 1 in]
            n280 = local read "Current Line"() -> (w1296:i32)
            n281 = Bundle By Name(cluster=w1298, "No. of command"=1003, "Boolean"=w1297, "No. of line"=w1296, "Status"="Pause" ("Sequence status")) -> (w1293:T3)
            n282 = Enqueue Element At Opposite End(queue=w1300, element=w1293, error in (no error)=w1299) -> (error out=w1295:errorcluster)  [unwired: 1 in, 2 out]
          }
          event "Program Stop": Value Change {
            n283 = event-data() -> ("NewVal"=w1306:bool)  [unwired: 1 in]
            n284 = Bundle By Name(cluster=w1305, "No. of command"=1005) -> (w1303:T3)
            n285 = Enqueue Element At Opposite End(queue=w1301, element=w1303, error in (no error)=w1302) -> (error out=w1307:errorcluster)  [unwired: 1 in, 2 out]
          }
          event "help": Value Change {
            n286 = event-data() -> ()  [unwired: 1 in, 1 out]
            n287 = Bundle By Name(cluster=w1313, "No. of command"=1006) -> (w1311:T3)
            n288 = Enqueue Element At Opposite End(queue=w1309, element=w1311, error in (no error)=w1310) -> (error out=w1314:errorcluster)  [unwired: 1 in, 2 out]
          }
          event Application Instance Close? {
            n289 = event-data() -> ()  [unwired: 1 in, 5 out]
            n290 = event-data("SilentShutdown"=TRUE) -> ()  [unwired: 1 in, 1 out]
          }
          event "sequence utility": Value Change {
            # "If true, current sequence and file path will be exported."
            n291 = event-data() -> ("CtlRef"=w1326:refnum<vi>)  [unwired: 1 in, 5 out]
            n292 = property on="Sequence" class="LstBox (strict)"() -> ("Item Names"=w1320:string[])  [unwired: 2 in, 2 out]
            n293 = property class="Bool (strict)"(reference=w1326, error in=w1325, "Value"=FALSE) -> (error out=w1324:errorcluster)  [unwired: 1 out]
            n294 = local read "Path"() -> (w1321:path)
            n295 = call "sequence utility.vi"("sequence in"=w1320, "error in (no error)"=w1324, "sequence path"=w1321, "platform"=w1328, "export?"=TRUE) -> ("error out"=w1323:errorcluster, "changed sequence"=w1318:string[], "do not update seq."=w1319:bool)  [unwired: 4 in]
            n296 = case shown="False" w1319 {
              tunnel: w1318 -> [w1329 _]
              frame False {
                n297 = property on="Sequence" class="LstBox (strict)"("Item Names"=w1329) -> ()  [unwired: 2 in, 2 out]
              }
              frame True {
              }
            }
          }
          event "exec window": Value Change {
            n298 = event-data() -> ("CtlRef"=w1346:refnum<vi>)  [unwired: 1 in, 5 out]
            n299 = case shown="0, Default" w1330 {
              tunnel: ["Monovu subvis/MonoVu_exec window.vi" ("name or relative path") "Monovu subvis\\MonoVu_exec window.vi" ("name or relative path")] -> w1342
              frame 0, Default {
              }
              frame 1 {
              }
            }
            n300 = property class="Bool (strict)"(reference=w1346, error in=w1345, "Value"=FALSE) -> (error out=w1344:errorcluster)  [unwired: 1 out]
            n301 = Current VI's Path() -> (path=w1338:path)
            n302 = Strip Path(path=w1338) -> (stripped path=w1337:path)  [unwired: 1 out]
            n303 = Build Path(base path=w1337, name or relative path=w1342) -> (appended path=w1341:path)
            n304 = Open VI Reference(vi path=w1341) -> (vi reference=w1340:refnum<vi>, error out=w1339:errorcluster)  [unwired: 5 in]
            n305 = invoke class="VI" method="FP.Open"(reference=w1340, error in=w1339) -> (reference out=w1336:refnum<vi>, error out=w1333:errorcluster)  [unwired: 3 in, 3 out]
            n306 = invoke class="VI" method="Run VI"(reference=w1336, error in=w1333, "Wait until done"=FALSE ("Wait Until Done")) -> (reference out=w1334:refnum<vi>, error out=w1332:errorcluster)  [unwired: 2 in, 3 out]
            n307 = Close Reference(reference=w1334, error in (no error)=w1332) -> (error out=→"error out":errorcluster)
          }
        }
        n308 = local write "loop stop"(w473) -> ()
      }
      n309 = while {
        shift-right: [w72] -> _
        shift-left: w41 -> [w73]
        tunnel: w36 -> [w71]
        tunnel: w40 -> [w70]
        tunnel: w39 -> [w69]
        tunnel: [w51] -> w33
        tunnel: w38 -> [w62]
        tunnel: w37 -> [w67]
        i -> [w58]
        stop <- w78 stop-if-true
        # "Message_Handler"
        n310 = Dequeue Element(queue=w71, error in (no error)=w70) -> (queue out=w76:refnum<queue>, element=w75:T3, error out=w77:errorcluster)  [unwired: 1 in, 1 out]
        n311 = Unbundle By Name(w75) -> ("No. of command"=w74:i32, "Subsequence"=w61:string[], "No. of line"=w44:i32)
        "macro line" <- w44
        n312 = Array Size(array=w61) -> (size(s)=w63:i32)
        n313 = case shown="1" w63 {
          tunnel: w61 -> [_ w89]
          tunnel: [w80 w84] -> w45
          tunnel: [w81 w87] -> w59
          tunnel: w44 -> [w81 w83]
          tunnel: [w80 w82] -> w47
          frame 0, Default {
            (unwired) FALSE ("Visible")
            w80 = ""
          }
          frame 1 {
            (unwired) TRUE ("Visible")
            n314 = Number To Decimal String(number=w83) -> (decimal integer string=w85:string)  [unwired: 1 in]
            n315 = local read "macro cmd no"() -> (w87:i32)
            n316 = Index Array(array=w89, index=0) -> (element=w82:string)
            n317 = Concatenate Strings(w82, w85, "\n") -> (w84:string)
          }
        }
        n318 = case shown="1001" w74 {
          tunnel: [_ _ _ _ _ _ _ _ _ _ _ _ _ _ _ _ FALSE _ _ _ _ TRUE _ _ _] -> w78
          tunnel: w77 -> [w96 w111 w124 w136 w148 w160 w176 w192 w204 w216 w227 w237 w251 w274 w304 w315 w323 w350 w384 w399 w422 w429 _ w450 w471]
          tunnel: [w90 w102 w114 w127 w139 w151 w163 w185 w195 w207 w220 w232 w242 w261 w294 w308 w320 w340 w380 w390 w403 w429 _ w441 w464] -> w68
          tunnel: w75 -> [w101 w105 w120 w132 w143 w157 w174 w182 w202 w214 w228 w240 w249 w256 w300 w316 _ _ _ _ w409 _ _ _ w468]
          tunnel: w76 -> [w100 w108 w121 w133 w147 w158 w177 w190 w201 w213 w229 w241 w252 w262 w301 w317 _ w348 w385 w400 w423 _ _ w461 w469]
          tunnel: w73 -> [w97 w112 w125 w137 w150 w161 w178 w193 w206 w218 w231 w235 w254 w276 w306 w319 w334 w343 w389 w397 w426 w430 w436 w451 w472]
          tunnel: [w94 w109 w123 w135 w149 w159 w175 w191 w205 w217 w230 w234 w253 w275 w305 w318 w326 w342 w388 w398 w425 w430 w436 w452 w470] -> w72
          tunnel: w69 -> [_ _ _ _ _ _ _ _ _ _ _ _ _ _ _ _ _ _ _ _ _ _ _ _ _]
          tunnel: w62 -> [_ _ _ _ _ _ _ _ _ _ _ _ _ _ _ _ _ _ _ _ _ _ _ _ _]
          tunnel: w67 -> [_ _ _ _ _ _ _ _ _ _ _ _ _ _ _ _ _ w336 _ _ _ _ _ w447 _]
          tunnel: [w91 w103 w116 w128 w140 w152 w165 w187 w197 w209 w222 w233 w245 w260 w302 w310 0 ("No. of line") w341 w386 w401 w417 0 ("No. of line") _ _ w466] -> w65
          tunnel: [w98 w113 w126 w138 w144 w154 w172 _ w198 w210 w224 w238 w246 _ w303 w312 "Idle" ("Status") "Idle or Waiting for the command complete" ("Status") "Pause" ("Status") "Idle" ("Status") "Skip" ("Sequence status") "Program Close" ("Sequence status") _ _ _] -> w64
          tunnel: FALSE ("Use LS336Panel.vi") -> [_ w104 _ _ w141 _ _ _ _ _ _ _ _ _ _ _ _ _ _ _ _ _ _ _ _]
          tunnel: "Magnet PS" -> [w92 _ _ _ _ w153 _ _ _ _ _ _ _ _ _ _ _ _ _ _ _ _ _ _ _]
          tunnel: w59 -> [w91 w103 w116 w128 w140 w152 w165 w187 w197 w209 w222 w233 w245 w260 w302 w310 _ _ _ _ _ _ _ _ w466]
          tunnel: [w90 w102 w114 w127 w139 w151 w162 w185 w194 _ w219 w232 w244 w261 w296 w307 w320 w337 w380 w390 w403 w429 errorcluster {"status"=FALSE, "code"=0, "source"=""} ("error out") w440 w464] -> w49
          tunnel: w47 -> [_ _ _ _ _ _ _ _ _ _ _ _ _ _ _ _ _ _ _ _ _ _ _ w439 _]
          tunnel: w45 -> [_ _ _ _ _ _ _ _ _ _ _ _ _ w259 _ _ _ _ _ _ _ _ _ _ _]
          frame 0 {
            # "Set Field"
            n319 = call "Start_Initial.vi"("error in (no error)"=w96, "Reference"=w97) -> ("error out"=w95:errorcluster, "dup Reference"=w94:T5)  [unwired: 8 in]
            n320 = call "Set_Field.vi"("Magnet PS"=w92, "error in (no error)"=w95, "Command_message_in"=w101, "Command_queue_in"=w100) -> ("error out"=w90:errorcluster, "Command_message_out"=w99:T4)  [unwired: 5 in, 1 out]
            n321 = Wait (ms)(milliseconds to wait=u32 100) -> ()  [unwired: 1 out]
            n322 = Unbundle By Name(w99) -> ("Status"=w98:string)
          }
          frame 1 {
            # "Set Temp"
            n323 = call "Start_Initial.vi"("error in (no error)"=w111, "Reference"=w112) -> ("error out"=w110:errorcluster, "dup Reference"=w109:T5)  [unwired: 8 in]
            n324 = call "Set_Temp.vi"("LS336FrontPanel.vi"=w104, "error in (no error)"=w110, "Message_command_in"=w105, "Command_queue_in"=w108) -> ("error out"=w102:errorcluster, "Message_command_out"=w107:T4)  [unwired: 6 in]
            n325 = Wait (ms)(milliseconds to wait=u32 100) -> ()  [unwired: 1 out]
            n326 = Unbundle By Name(w107) -> ("Status"=w113:string)
          }
          frame 2 {
            # "Start DAQ"
            n327 = control-ref of="NML Data Acquisition VI"() -> (w118:refnum<vi>)
            n328 = call "Start_Initial.vi"("error in (no error)"=w124, "Reference"=w125) -> ("error out"=w122:errorcluster, "dup Reference"=w123:T5)  [unwired: 8 in]
            n329 = local read "platform"() -> (w115:u16)
            n330 = call "Start_DAQ.vi"("platform"=w115, "error in (no error)"=w122, "Command_Queue_in"=w121, "Command_message_in"=w120, "DAQ in"=w118) -> ("error out"=w114:errorcluster, "Command_message_out"=w119:T4)  [unwired: 5 in]
            n331 = Unbundle By Name(w119) -> ("Status"=w126:string)
            n332 = Wait (ms)(milliseconds to wait=u32 100) -> ()  [unwired: 1 out]
          }
          frame 3 {
            # "Stop DAQ"
            n333 = control-ref of="NML Data Acquisition VI"() -> (w130:refnum<vi>)
            n334 = call "Start_Initial.vi"("error in (no error)"=w136, "Reference"=w137) -> ("error out"=w134:errorcluster, "dup Reference"=w135:T5)  [unwired: 8 in]
            n335 = call "Stop_DAQ.vi"("error in (no error)"=w134, "Command_Queue_in"=w133, "Command_message_in"=w132, "DAQ in"=w130) -> ("error out"=w127:errorcluster, "Command_message_out"=w131:T4)  [unwired: 6 in]
            n336 = Unbundle By Name(w131) -> ("Status"=w138:string)
            n337 = Wait (ms)(milliseconds to wait=u32 100) -> ()  [unwired: 1 out]
          }
          frame 4 {
            # "Wait for Temperature"
            n338 = call "Start_Initial.vi"("error in (no error)"=w148, "Reference"=w150) -> ("error out"=w146:errorcluster, "dup Reference"=w149:T5)  [unwired: 8 in]
            n339 = Wait (ms)(milliseconds to wait=u32 100) -> ()  [unwired: 1 out]
            n340 = call "Wait_for_Temp.vi"("LS336FrontPanel.vi"=w141, "error in (no error)"=w146, "Message_command in"=w143, "Command Queue"=w147) -> ("error out"=w139:errorcluster, "dup Message_command"=w145:T4)  [unwired: 6 in]
            n341 = Unbundle By Name(w145) -> ("Status"=w144:string)
          }
          frame 5 {
            # "Wait for Field Stable"
            n342 = call "Start_Initial.vi"("error in (no error)"=w160, "Reference"=w161) -> ("error out"=w156:errorcluster, "dup Reference"=w159:T5)  [unwired: 8 in]
            n343 = call "Wait_for_field_stable.vi"("Magnet PS"=w153, "error in (no error)"=w156, "Message_command in"=w157, "Command_Queue"=w158) -> ("error out"=w151:errorcluster, "Message_command out"=w155:T4)  [unwired: 6 in]
            n344 = Unbundle By Name(w155) -> ("Status"=w154:string)
          }
          frame 7 {
            # "Remarks"
            n345 = call "Start_Initial.vi"("error in (no error)"=w176, "Reference"=w178) -> ("error out"=w173:errorcluster, "dup Reference"=w175:T5)  [unwired: 8 in]
            n346 = call "Library2.vi"("Message_command_in"=w174, "error in (no error)"=w173) -> ("Message_command out"=w167:T4, "error out"=w164:errorcluster)  [unwired: 7 in]
            n347 = Unbundle By Name(w167) -> ("Sequence_History"=w171:string, "Status"=w170:string)
            n348 = Concatenate Strings(w171, w170, "\r") -> (w168:string)
            n349 = Bundle By Name(cluster=w167, "Sequence_History"=w168) -> (w166:T4)
            n350 = call "go_to_next_line.vi"("error in (no error)"=w164, "Message_command in"=w166, "Command Queue in"=w177) -> ("error out"=w163:errorcluster)  [unwired: 7 in, 1 out]
            n351 = Unbundle By Name(w167) -> ("Status"=w172:string)
            n352 = Merge Errors(w164, w163) -> (w162:errorcluster)
          }
          frame 8 {
            # "Run Macro"
            n353 = call "Start_Initial.vi"("error in (no error)"=w192, "Reference"=w193) -> ("error out"=w189:errorcluster, "dup Reference"=w191:T5)  [unwired: 8 in]
            n354 = Unbundle By Name(w182) -> ("Status"=w181:string)
            n355 = Unbundle By Name(w182) -> ("No. of line"=w188:i32)
            n356 = Match Pattern(string=w181, regular expression="Run Macro ") -> (after substring=w179:string)  [unwired: 1 in, 3 out]
            n357 = Concatenate Strings("Macro Started: " ("input"), w179) -> (w183:string)
            n358 = property on="macro cmd no" class="DigNum (strict)"("Value"=w188) -> ()  [unwired: 2 in, 2 out]
            n359 = call "RunMacro.vi"("submacro"=FALSE, "error in (no error)"=w189, "Message_command"=w182, "queue"=w190) -> ("error out"=w185:errorcluster)  [unwired: 5 in, 2 out]
            n360 = call "write to log file.vi"("input"=w183) -> ()  [unwired: 9 in, 1 out]
          }
          frame 9 {
            # "Run VI"
            n361 = call "Start_Initial.vi"("error in (no error)"=w204, "Reference"=w206) -> ("error out"=w203:errorcluster, "dup Reference"=w205:T5)  [unwired: 8 in]
            n362 = call "Run_VI.vi"("error in (no error)"=w203, "Message_command_in"=w202, "Command Queue in"=w201) -> ("error out"=w196:errorcluster, "Message_command out"=w199:T4, "Command Queue out"=w200:T6)  [unwired: 5 in, 1 out]
            n363 = call "go_to_next_line.vi"("error in (no error)"=w196, "Message_command in"=w199, "Command Queue in"=w200) -> ("error out"=w195:errorcluster)  [unwired: 7 in, 1 out]
            n364 = Unbundle By Name(w199) -> ("Status"=w198:string)
            n365 = Merge Errors(w196, w195) -> (w194:errorcluster)
          }
          frame 10 {
            # "Error reporting disabled\nfor Abort.vi"
            # "Abort VI"
            n366 = call "Start_Initial.vi"("error in (no error)"=w216, "Reference"=w218) -> ("error out"=w215:errorcluster, "dup Reference"=w217:T5)  [unwired: 8 in]
            n367 = call "Abort_VI.vi"("error in (no error)"=w215, "Message_command_in"=w214, "Command Queue in"=w213) -> ("error out"=w208:errorcluster, "Message_command out"=w211:T4, "Command Queue out"=w212:T6)  [unwired: 5 in, 1 out]
            n368 = call "go_to_next_line.vi"("error in (no error)"=w208, "Message_command in"=w211, "Command Queue in"=w212) -> ("error out"=w207:errorcluster)  [unwired: 7 in, 1 out]
            n369 = Unbundle By Name(w211) -> ("Status"=w210:string)
          }
          frame 11 {
            # "Set Device"
            n370 = call "Start_Initial.vi"("error in (no error)"=w227, "Reference"=w231) -> ("error out"=w226:errorcluster, "dup Reference"=w230:T5)  [unwired: 8 in]
            n371 = call "Run_Device.vi"("error in (no error)"=w226, "Message_command"=w228, "Command Queue"=w229) -> ("error out"=w221:errorcluster, "dup Message_command"=w223:T4, "dup Command Queue"=w225:T6)  [unwired: 6 in]
            n372 = call "go_to_next_line.vi"("error in (no error)"=w221, "Message_command in"=w223, "Command Queue in"=w225) -> ("error out"=w220:errorcluster)  [unwired: 7 in, 1 out]
            n373 = Unbundle By Name(w223) -> ("Status"=w224:string)
            n374 = Merge Errors(w220, w221) -> (w219:errorcluster)
          }
          frame 12 {
            # "Wait for"
            n375 = call "Start_Initial.vi"("error in (no error)"=w237, "Reference"=w235) -> ("error out"=w236:errorcluster, "dup Reference"=w234:T5)  [unwired: 8 in]
            n376 = call "Wait_for.vi"("error in (no error)"=w236, "Message_command in"=w240, "Command Queue"=w241) -> ("error out"=w232:errorcluster, "dup Message_command"=w239:T4)  [unwired: 7 in]
            n377 = Unbundle By Name(w239) -> ("Status"=w238:string)
          }
          frame 13 {
            # "Set Parameter"
            n378 = call "Start_Initial.vi"("error in (no error)"=w251, "Reference"=w254) -> ("error out"=w250:errorcluster, "dup Reference"=w253:T5)  [unwired: 8 in]
            n379 = call "Set_Parameters.vi"("error in (no error)"=w250, "Message_command In"=w249, "Command Queue In"=w252) -> ("error out"=w243:errorcluster, "Message_command Out"=w247:T4, "Command Queue out"=w248:T6)  [unwired: 6 in]
            n380 = Unbundle By Name(w247) -> ("Status"=w246:string)
            n381 = call "go_to_next_line.vi"("error in (no error)"=w243, "Message_command in"=w247, "Command Queue in"=w248) -> ("error out"=w242:errorcluster)  [unwired: 7 in, 1 out]
            n382 = Merge Errors(w242, w243) -> (w244:errorcluster)
          }
          frame 14 {
            # "Wait for any VI value"
            n383 = call "Start_Initial.vi"("error in (no error)"=w274, "Reference"=w276) -> ("error out"=w273:errorcluster, "dup Reference"=w275:T5)  [unwired: 8 in]
            n384 = local write "loop stop"(FALSE ("loop stop")) -> ()
            n385 = call "WaitForAnyVI_initialize.vi"("Message_command In"=w256) -> ("current time"=w265:timestamp, "parameters"=w267:string[], "vi reference"=w271:refnum<vi>, "application reference"=w272:refnum<vi>)  [unwired: 7 in]
            n386 = while {
              shift-right: [w292] -> w264
              shift-left: w273 -> [w293]
              shift-right: [w291] -> w268
              shift-left: w272 -> [w288]
              shift-right: [w290] -> w269
              shift-left: w271 -> [w287]
              tunnel: w267 -> [w289]
              shift-right: [w284] -> _
              shift-left: u32 0 ("millisecond timer value") -> [w286]
              tunnel: w265 -> [w285]
              tunnel: w259 -> [w283]
              tunnel: [w281] -> w257
              stop <- w279 stop-if-true
              n387 = call "WaitForAnyVI.vi"("application reference"=w288, "vi reference"=w287, "Initial Time"=w285, "parameters"=w289, "error in (no error)"=w293, "counter in"=w286) -> ("counter out"=w284:i32, "status"=w281:string, "application reference out"=w291:refnum<vi>, "Done"=w278:bool, "vi reference out"=w290:refnum<vi>, "error out"=w292:errorcluster)  [unwired: 4 in]
              n388 = Concatenate Strings(w283, w281) -> (w282:string)
              n389 = local write "Sequence Status"(w282) -> ()
              n390 = Or(x=w278, y="loop stop") -> (x .or. y?=w279:bool)
              n391 = Wait (ms)(milliseconds to wait="looped command interval (ms)") -> ()  [unwired: 1 out]
            }
            n392 = Close Reference(reference=w269, error in (no error)=w264) -> (error out=w270:errorcluster)
            n393 = Bundle By Name(cluster=w256, "Status"=w257) -> (w258:T3)
            n394 = Close Reference(reference=w268, error in (no error)=w270) -> (error out=w263:errorcluster)
            n395 = call "go_to_next_line.vi"("error in (no error)"=w263, "Message_command in"=w258, "Command Queue in"=w262) -> ("error out"=w261:errorcluster)  [unwired: 7 in, 1 out]
          }
          frame 15 {
            # "Write to VISA"
            n396 = call "Start_Initial.vi"("error in (no error)"=w304, "Reference"=w306) -> ("error out"=w299:errorcluster, "dup Reference"=w305:T5)  [unwired: 8 in]
            n397 = call "Write2VISA.vi"("error in (no error)"=w299, "Message_command In"=w300, "Command Queue In"=w301) -> ("error out"=w295:errorcluster, "Message_command Out"=w297:T4, "Command Queue out"=w298:T6)  [unwired: 6 in]
            n398 = call "go_to_next_line.vi"("error in (no error)"=w295, "Message_command in"=w297, "Command Queue in"=w298) -> ("error out"=w294:errorcluster)  [unwired: 7 in, 1 out]
            n399 = Unbundle By Name(w297) -> ("Status"=w303:string)
            n400 = Merge Errors(w294, w295) -> (w296:errorcluster)
          }
          frame 16 {
            # "Sweep"
            n401 = call "Start_Initial.vi"("error in (no error)"=w315, "Reference"=w319) -> ("error out"=w314:errorcluster, "dup Reference"=w318:T5)  [unwired: 8 in]
            n402 = call "Sweep_device.vi"("error in (no error)"=w314, "Message_command"=w316, "Command Queue"=w317) -> ("error out"=w309:errorcluster, "dup Message_command"=w311:T4, "dup Command Queue"=w313:T6)  [unwired: 6 in]
            n403 = call "go_to_next_line.vi"("error in (no error)"=w309, "Message_command in"=w311, "Command Queue in"=w313) -> ("error out"=w308:errorcluster)  [unwired: 7 in, 1 out]
            n404 = Unbundle By Name(w311) -> ("Status"=w312:string)
            n405 = Merge Errors(w308, w309) -> (w307:errorcluster)
          }
          frame 1000, Default {
            # "Program Initialize"
            n406 = control-ref of="NML Data Acquisition VI"() -> (w328:refnum<vi>)
            n407 = control-ref of="Sequence_Stop"() -> (w331:refnum<vi>)
            n408 = control-ref of="Run Sequence"() -> (w333:refnum<vi>)
            n409 = control-ref of="Program Stop"() -> (w329:refnum<vi>)
            n410 = control-ref of="Pause Button"() -> (w332:refnum<vi>)
            n411 = control-ref of="Skip Button"() -> (w330:refnum<vi>)
            n412 = control-ref of="Sequence"() -> (w321:refnum<vi>)
            n413 = Bundle By Name(cluster=w334, "Sequence_Run"=w333, "Sequence_Pause"=w332, "Sequence_Stop"=w331, "Sequence_Skip"=w330, "Program Stop"=w329, "Sequence"=w321, "NML Data Acquisition VI"=w328) -> (w327:T5)
            n414 = call "Program_initial.vi"("error in (no error)"=w323, "Reference"=w327) -> ("error out"=w320:errorcluster, "dup Reference"=w326:T5)  [unwired: 8 in]
          }
          frame 1001 {
            # "Run Sequence"
            n415 = Unbundle By Name(w343) -> ("Sequence"=w345:refnum<vi>)
            n416 = local read "error\ncheck"() -> (w335:bool)
            n417 = call "Sequence_Message_initial_line.vi"("reference"=w345, "error check?"=w335, "error in (no error)"=w350) -> ("Number of begin"=w346:u16, "Run?"=w349:bool, "error out"=w347:errorcluster)  [unwired: 5 in]
            n418 = case shown="True" w349 {
              tunnel: w348 -> [w361 w374]
              tunnel: w347 -> [w352 w366]
              tunnel: [w351 w362] -> w340
              tunnel: w336 -> [w354 w377]
              tunnel: w346 -> [_ w367]
              tunnel: [w357 w373] -> _
              tunnel: w345 -> [_ w371]
              tunnel: w343 -> [w360 w370]
              tunnel: [w360 w368] -> w342
              tunnel: [w353 w367] -> w341
              tunnel: [w352 w363] -> w339
              tunnel: [w351 w362] -> w338
              frame False {
                n419 = Unbundle By Name(w354) -> ("No. of line"=w353:i32)
                n420 = Bundle By Name(cluster=w354, "No. of command"=1000, "No. of line"=w353) -> (w355:T3)
                n421 = Flush Queue(queue=w361, error in (no error)=w352) -> (queue out=w359:refnum<queue>, error out=w358:errorcluster)  [unwired: 1 out]
                n422 = Enqueue Element(queue=w359, element=w355, error in (no error)=w358) -> (queue out=w357:refnum<queue>, error out=w351:errorcluster)  [unwired: 1 in, 1 out]
              }
              frame True {
                n423 = Get Date/Time In Seconds() -> (seconds since 1Jan1904=w372:timestamp)
                n424 = Bundle By Name(cluster=w377, "No. of line"=w367, "Initial Time"=w372, "Sequence Ref."=w371) -> (w376:T3)
                n425 = call "Library2.vi"("Message_command_in"=w376, "error in (no error)"=w366) -> ("Message_command out"=w375:T4, "error out"=w363:errorcluster)  [unwired: 7 in]
                n426 = case shown="False" "override command error" {
                  tunnel: [w378 errorcluster {"status"=FALSE, "code"=0, "source"=""} ("error in (no error)")] -> w364
                  tunnel: w363 -> [w378 _]
                  frame False {
                  }
                  frame True {
                  }
                }
                n427 = Enqueue Element(queue=w374, element=w375, error in (no error)=w364) -> (queue out=w373:refnum<queue>, error out=w369:errorcluster)  [unwired: 1 in, 1 out]
                n428 = call "Start_Initial.vi"("error in (no error)"=w369, "Reference"=w370) -> ("error out"=w362:errorcluster, "dup Reference"=w368:T5)  [unwired: 8 in]
              }
            }
            n429 = Merge Errors(w339, w338) -> (w337:errorcluster)
          }
          frame 1002 {
            # "Sequence_Pause"
            n430 = Flush Queue(queue=w385, error in (no error)=w384) -> (error out=w383:errorcluster)  [unwired: 2 out]
            n431 = call "Pause_Initial.vi"("error in (no error)"=w383, "Blinking"=TRUE, "Reference"=w389) -> ("error out"=w380:errorcluster, "dup Reference"=w388:T5)  [unwired: 7 in]
            n432 = call "write to log file.vi"("input"="!!! Pause button pressed !!!") -> ()  [unwired: 9 in, 1 out]
            n433 = local read "Current Line"() -> (w386:i32)
          }
          frame 1003 {
            # "Sequence_Stop"
            n434 = local read "Current Line"() -> (w393:i32)
            n435 = Flush Queue(queue=w400, error in (no error)=w399) -> (error out=w396:errorcluster)  [unwired: 2 out]
            n436 = property on="Sequence" class="LstBox (strict)"() -> ("Item Names"=w392:string[])  [unwired: 2 in, 2 out]
            n437 = Index Array(array=w392, index=w393) -> (element=w394:string)
            n438 = Concatenate Strings("!!! Stop button pressed !!!" ("input"), w394) -> (w395:string)
            n439 = call "write to log file.vi"("input"=w395) -> ()  [unwired: 9 in, 1 out]
            n440 = local read "Current Line"() -> (w401:i32)
            n441 = call "Program_initial.vi"("error in (no error)"=w396, "Reference"=w397) -> ("error out"=w390:errorcluster, "dup Reference"=w398:T5)  [unwired: 8 in]
          }
          frame 1004 {
            # "1. skipped sequence is added in the log\n2. Checks if it is resulted from idle or not found command."
            # "Sequence_Skip"
            n442 = local read "Current Line"() -> (w411:i32)
            n443 = Get Date/Time In Seconds() -> (seconds since 1Jan1904=w419:timestamp)
            n444 = control-ref of="Sequence"() -> (w418:refnum<vi>)
            n445 = Flush Queue(queue=w423, error in (no error)=w422) -> (queue out=w421:refnum<queue>, error out=w420:errorcluster)  [unwired: 1 out]
            n446 = property on="Sequence" class="LstBox (strict)"() -> ("Item Names"=w412:string[])  [unwired: 2 in, 2 out]
            n447 = Bundle By Name(cluster=w409, "No. of line"=w411, "Initial Time"=w419, "Sequence Ref."=w418) -> (w416:T3)
            n448 = call "Start_Initial.vi"("error in (no error)"=w420, "Reference"=w426) -> ("error out"=w424:errorcluster, "dup Reference"=w425:T5)  [unwired: 8 in]
            n449 = Unbundle By Name(w409) -> ("Status"=w407:string)
            n450 = Index Array(array=w412, index=w411) -> (element=w410:string)
            n451 = Concatenate Strings("!!! SKIP !!! " ("string"), w410) -> (w404:string)
            n452 = Equal?(x=w407, y="Unidentified command. Skipped" ("Status")) -> (x = y?=w406:bool)
            n453 = case shown="True" w406 {
              tunnel: [w427 "doo nott write to log"] -> w405
              tunnel: w404 -> [w427 _]
              frame False {
              }
              frame True {
              }
            }
            n454 = Bundle By Name(cluster=w416, "Status"=w405) -> (w415:T3)
            n455 = Unbundle By Name(w415) -> ("No. of line"=w417:i32)
            n456 = call "go_to_next_line.vi"("error in (no error)"=w424, "Message_command in"=w415, "Command Queue in"=w421) -> ("error out"=w403:errorcluster)  [unwired: 7 in, 1 out]
          }
          frame 1005 {
            # "Program Stop"
          }
          frame 1006 {
            # "Open html help document"
            n457 = call-poly <vilib>:"Open HTML Report in Browser.vi"("URL"="https://opsserver.magnet.fsu.edu/wiki/pages/j6n0H6L5/MonoVuvi_Instruction.html") -> ()  [unwired: 13 in, 2 out]
          }
          frame 1007 {
            # "1. Delete queues of command lines in the subsequences\n2. Returns to the next line of the main sequences."
            # "END SUBsequence"
            n458 = Match Pattern(string=w439, regular expression=",  line #: " ("string")) -> (before substring=w437:string)  [unwired: 1 in, 3 out]
            n459 = Get Date/Time In Seconds() -> (seconds since 1Jan1904=w458:timestamp)
            n460 = Flush Queue(queue=w461, error in (no error)=w450) -> (queue out=w453:refnum<queue>, error out=w449:errorcluster)  [unwired: 1 out]
            n461 = Unbundle By Name(w451) -> ("Sequence"=w457:refnum<vi>)
            n462 = property on="macro cmd no" class="DigNum (strict)"() -> ("Value"=w460:i32)  [unwired: 2 in, 2 out]
            n463 = local read "override command error"() -> (w446:bool)
            n464 = Increment(x=w460) -> (x+1=w459:i32)
            n465 = Bundle By Name(cluster=w447, "No. of line"=w459, "Initial Time"=w458, "Sequence Ref."=w457, "Subsequence"=string[] []) -> (w456:T3)
            n466 = call "Library2.vi"("Message_command_in"=w456, "error in (no error)"=w449) -> ("Message_command out"=w454:T4, "error out"=w442:errorcluster)  [unwired: 7 in]
            n467 = case shown="True" w446 {
              tunnel: [w462 errorcluster {"status"=FALSE, "code"=0, "source"=""} ("error in (no error)")] -> w445
              tunnel: w442 -> [w462 _]
              frame False {
              }
              frame True {
              }
            }
            n468 = Concatenate Strings("Macro Ended: " ("input"), w437) -> (w443:string)
            n469 = Enqueue Element(queue=w453, element=w454, error in (no error)=w445) -> (error out=w455:errorcluster)  [unwired: 1 in, 2 out]
            n470 = call "write to log file.vi"("input"=w443) -> ()  [unwired: 9 in, 1 out]
            n471 = call "Start_Initial.vi"("error in (no error)"=w455, "Reference"=w451) -> ("error out"=w441:errorcluster, "dup Reference"=w452:T5)  [unwired: 8 in]
            n472 = Merge Errors(w442, w441) -> (w440:errorcluster)
          }
          frame 1008 {
            # "Nested submacros are unnested to make a single expanded macro (see\ncommand line 8)."
            # "SubMacro"
            n473 = call "Start_Initial.vi"("error in (no error)"=w471, "Reference"=w472) -> ("error out"=w467:errorcluster, "dup Reference"=w470:T5)  [unwired: 8 in]
            n474 = call "RunMacro.vi"("submacro"=TRUE, "error in (no error)"=w467, "Message_command"=w468, "queue"=w469) -> ("error out"=w464:errorcluster)  [unwired: 5 in, 2 out]
          }
        }
        "Current Line" <- w65
        n475 = Unbundle By Name(w49) -> ("code"=w56:i32)
        n476 = Concatenate Strings(w45, w64) -> (→"Sequence Status":string)
        n477 = Not Equal To 0?(x=w56) -> (x != 0?=w48:bool)
        n478 = call <vilib>:"Clear Errors.vi"("error in (no error)"=w68) -> ("error out"=w51:errorcluster)  [unwired: 5 in, 1 out]
        n479 = property on="Error/\nwarning?" class="Bool (strict)"() -> ("Value"=w52:bool)  [unwired: 2 in, 2 out]
        n480 = property on="reset error indicator" class="Bool"("Visible"=w52) -> ()  [unwired: 2 in, 2 out]
        n481 = Or(x=w52, y=w48) -> (x .or. y?=w54:bool)
        n482 = Not(x="reset error indicator") -> (.not. x?=w53:bool)
        n483 = And(x=w54, y=w53) -> (x .and. y?=→"Error/\nwarning?":bool)
        n484 = case shown="True" w48 {
          tunnel: w49 -> [_ w79]
          frame False {
          }
          frame True {
            "latest error" <- w79
          }
        }
        n485 = Wait Until Next ms Multiple(millisecond multiple="wait (ms)") -> ()  [unwired: 1 out]
        "execution count" <- w58
      }
      n486 = Merge Errors(w35, w33) -> (w42:errorcluster)
    }
    frame Error {
    }
  }
  n487 = local write "sequence utility"(w2) -> ()
  n488 = local write "exec window"(w2) -> ()
  n489 = Unregister For Events(event registration refnum=w14, error in=w13) -> (error out=w12:errorcluster)
  n490 = Release Queue(queue=w15, error in (no error)=w12) -> ()  [unwired: 1 in, 3 out]
  "Buffer History" <- w5
  "Buffer Edit" <- w5
